vi "MoD Main-Optimize - HPLC RedAm_72117.vi"() -> ()   [LabVIEW 2015]
uses:
  <vilib>/silver_ctls/ArrayMatrixCluster/Real Matrix NI_Silver.ctl
  <vilib>/ni845x/ni845x.llb/ni845xControl.ctl
  <vilib>/MakerHub/LINX/Public/Peripherals/Analog/Analog Read 1 Chan.vi
  <vilib>/MakerHub/LINX/Public/Peripherals/Analog/Analog Read N Chans.vi
  <vilib>/MakerHub/LINX/Public/Peripherals/Digital/Digital Write 1 Chan.vi
  <vilib>/MakerHub/LINX/Private/Local IO/LinxAnalogRead.vi
  <vilib>/MakerHub/LINX/Public/Utilities/Check Channel.vi
  <vilib>/MakerHub/LINX/Public/Peripherals/Digital/Digital Write N Chans.vi
  <vilib>/MakerHub/LINX/Private/Local IO/LinxDigitalWrite.vi
  <vilib>/addons/control/pid/pid.llb/PID Control Input Filter (DBL).vi
  <vilib>/MakerHub/LINX/Private/Utilties/Generate Error.vi
  <vilib>/addons/control/pid/autopid.llb/PID Online Autotuning (Relay Feedback).vi
  <vilib>/Analysis/Matrix/Numeric/Conversions/Array To Matrix - RA2.vi
  <vilib>/ni845x/ni845x.llb/NI-845x Close Device Reference.vi
  <vilib>/addons/control/pid/NI_PID_autopid.lvlib
  <vilib>/addons/control/pid/NI_PID_pid.lvlib
  <vilib>/Analysis/Matrix/NI_Matrix.lvlib
  <vilib>/MakerHub/LINX/LMH-LINX.lvlib
  <instrlib>/Harvard Apparatus PHD Ultra Series/Harvard Apparatus PHD Ultra Series.lvlib
panel:
  out "running?":bool=TRUE
  out "new_reactor_volume":bool[](array[boolean])
  out "new_reactor_length":bool[](array[boolean])
  out "Phase_Sensor_voltage":dbl
  out "P_tot":dbl
  out "pause for ms":bool=TRUE
  out "stop_xl_write":bool=TRUE
  out "Num_exp_till_pause":i32
  out "Syringe_pump?":bool=TRUE
  out "System Error":bool=TRUE
  out "error out":errorcluster
  out "Pump setpoint(ul/min) 6":dbl format="%#_13g"
  out "Pump setpoint(ul/min) 5":dbl format="%#_13g"
  out "Pump setpoint(ul/min) 4":dbl format="%#_13g"
  out "Pump setpoint(ul/min) 3":dbl format="%#_13g"
  out "Pump setpoint(ul/min) 2":dbl format="%#_13g"
  out "Pump setpoint(ul/min) 1":dbl format="%#_13g"
  out "Volume (ul) 5":dbl format="%#_13g"
  out "Volume (ul) 4":dbl format="%#_13g"
  out "Volume (ul) 3":dbl format="%#_13g"
  out "Volume (ul) 2":dbl format="%#_13g"
  out "Volume (ul) 1":dbl format="%#_13g"
  in  "tau 5":dbl format="%#_13g"
  out "tau 4":dbl format="%#_13g"
  out "tau 3":dbl format="%#_13g"
  out "tau 2":dbl format="%#_13g"
  out "tau 1":dbl format="%#_13g"
  out "Reactor Length":dbl format="%#_13g"
  out "Flowrate Sensor 2":dbl format="%#_13g"
  out "Flowrate Sensor 1":dbl format="%#_13g"
  out "Pressure 2":dbl format="%#_13g"
  out "Pressure 1":dbl format="%#_13g"
  out "Temperature Control 5":bool=TRUE
  out "Temperature Control 4":bool=TRUE
  out "Temperature Control 3":bool=TRUE
  out "Temperature Control 2":bool=TRUE
  out "Temperature Control 1":bool=TRUE
  out "Temperature SP 5":dbl format="%#_g'C"
  out "Temperature SP 4":dbl format="%#_g'C"
  out "Temperature SP 3":dbl format="%#_g'C"
  out "Temperature SP 2":dbl format="%#_g'C"
  out "Temperature SP 1":dbl format="%#_g'C"
  in  "Bay Temperature 5":dbl
  in  "SSR Duration 5":dbl
  in  "SSR Duration 4":dbl
  in  "SSR Duration 3":dbl
  in  "SSR Duration 2":dbl
  in  "SSR Duration 1":dbl
  in  "Total Product Amount":dbl=1.0 format="%#_gml"
  out "Setup Error":bool=TRUE
  out "Error Message":string
  out "ID CTR":i32
  in  "Tab Control":T1(tab)
  out "Reagent pic 5":picture
  in  "reagent name 5":string
  out "Reagent Pic 4":picture
  in  "reagent name 4":string="Acetic Acid"
  out "Reagent Pic 3":picture
  in  "reagent  name 3":string="NaBH3CN"
  in  "Product name":string
  in  "reagent name 1":string="cyclohexylamine"
  out "Reagent Pic 1":picture
  in  "Vr5":dbl=45.6036 format="%#_guL"
  in  "Vr4":dbl format="%#_guL"
  in  "Vr3":dbl=45.6036 format="%#_guL"
  in  "Vr2":dbl format="%#_guL"
  in  "Vr1":dbl format="%#_guL"
  in  "System decide help Button":bool
  in  "Reaction Scheme Confirm":bool
  in  "Synthesis Route Array":string[][](array[string])=[["cyclohexylamine", ".1", "PhB(OH)2", "", "", ""], ["aldehyde + STD", ".1", "-", "-", "-", "-"], ["NaBH3CN", ".4", "-", "-", "-", "-"], ["Acetic Acid", "1", "-", "-", "-", "-"], ["", "", "-", "-", "-", "-"], ["", "", "-", "-", "-", "-"]]
  in  "System decide help Button 2":bool
  out "Setup Confirm":bool=TRUE
  in  "BAY 1":u16(ring)=1 items=["               Bypass", "         Heated Reactor", "    Small Heated Reator", "         Cooled Reactor", "      Packed Bed Reactor", "          Photo Reactor", "             Separator"]
  in  "BAY 5":u16(ring) items=["               Bypass", "         Heated Reactor", "    Small Heated Reactor", "         Cooled Reactor", "     Packed Bed Reactor", "         Photo Reactor", "             Separator"]
  in  "BAY 4":u16(ring) items=["                Bypass", "         Heated Reactor", "    Small Heated Reactor", "         Cooled Reactor", "     Packed Bed Reactor", "         Photo Reactor", "             Separator"]
  in  "BAY 3":u16(ring)=1 items=["               Bypass", "         Heated Reactor", "    Small Heated Reactor", "         Cooled Reactor", "     Packed Bed Reactor", "          Photo Reactor", "             Separator"]
  in  "BAY 2":u16(ring) items=["               Bypass", "         Heated Reactor", "    Small Heated Reactor", "         Cooled Reactor", "      Packed Bed Reactor", "          Photo Reactor", "             Separator"]
  out "Reagent Pic 2":picture
  out "Product Pic":picture
  in  "reagent name 2":string="benzylaldehyde"
  in  "reagent name 6":string
  out "Reagent Pic 6":picture
  in  "System Parameters Help Button":bool
  out "Setup Confirm 2":bool
  in  "System Parameters Confirm Button":bool
  in  "Bay Parameters":T2={"Bay 1 "={"Pump 1 Flowrate"=0.0, "optimize_temp"=TRUE, "optimize_tau"=TRUE, "Run at set flowrate"=FALSE, "Pump 2 Flowrate"=0.0, "Temperature Params"=[40.0, 100.0, 100.0], "pump params 1"=[43.0, 429.0, 325.0], "pump params 2"=[43.0, 429.0, 325.0], "Temperature"=0.0, "Run at set temperature"=FALSE}, "Bay 2 "={"Pump 3 Flowrate"=0.0, "optimize_temp"=FALSE, "optimize_tau"=TRUE, "Run at set flowrate"=FALSE, "Temperature Params"=[40.0, 100.0, 100.0], "Resisdence time params"=[38.03, 347.0, 650.0], "pump_at_ratio"=TRUE, "pump_num_ratio"=0.475, "Temperature"=0.0, "Run at set temperature"=FALSE}, "Bay 3 "={"Pump 4 Flowrate"=100.0, "optimize_temp"=FALSE, "optimize_tau"=FALSE, "Run at set flowrate"=FALSE, "Temperature Params"=[40.0, 100.0, 100.0], "Resisdence time params"=[3.8, 34.7, 0.0], "pump_at_ratio"=TRUE, "pump_num_ratio"=0.2, "Temperature "=100.0, "Run at set temperature"=TRUE}, "Bay 4 "={"Pump 5 Flowrate"=40.0, "Run at set flowrate"=FALSE, "optimize_temp"=FALSE, "optimize_tau"=FALSE, "Resisdence time params"=[10.0, 50.0, 225.0], "Temperature Params"=[40.0, 100.0, 80.0], "pump_at_ratio"=FALSE, "pump_num_ratio"=1.0, "Temperature"=0.0, "Run at set temperature"=FALSE}, "Bay 5 "={"Pump 6 Flowrate"=0.0, "Run at set flowrate"=FALSE, "optimize_temp"=FALSE, "optimize_tau"=FALSE, "Resisdence time params"=[1.0, 5.0, 0.0], "Temperature Params"=[0.0, 0.0, 0.0], "pump_at_ratio"=FALSE, "pump_num_ratio"=0.5, "Temperature"=0.0, "Run at set temperature"=FALSE}, "Excel File Name"="C:\\Users\\HPLC\\Dropbox (MIT)\\MoD Files\\Data\\RedAmin072117", "hplc File Name"="C:\\Chem32\\1\\Data\\MOD", "Matlab File"="C:\\Users\\HPLC\\Dropbox (MIT)\\MoD Files\\Data\\RedAmin072117", "Syringe for Pump 2?"=FALSE, "Num_conditons_per_wait"=2.0, "Continue from previous optimization?"=FALSE, "Total Number of Experiments 2"=15.0, "Hplc Wait time(min)"=10.0, "increas_decrease_hplc_peak"=TRUE, "Internal Standard?"=TRUE, "ISTD start"=8.0, "ISTD end"=10.0, "hplc_start"=1.75, "hplc_end"=3.0, "throughput_yield"=TRUE} {"Hplc Wait time(min)" format="%#_13g"; "Bay 5"."Temperature Params" format="%#_g'C"; "Bay 4"."Temperature Params" format="%#_g'C"; "Bay 3"."Temperature Params" format="%#_g'C"; "Bay 2"."Temperature Params" format="%#_g'C"; "Bay 1"."Temperature Params" format="%#_g'C"}
  out "System Confirm Not Clicked":string
  out "best_exp_num":dbl=1.0
  out "temperature_best":dbl[](array[numeric])
  out "Flowrates(ul/min)_best":dbl[](array[numeric])
  out "System Status":u16(ring)=2 caption="Sy" items=["System  Error", "System Running", "System Standby"]
  out "Current Experiment":dbl=1.0
  out "Total Number of Experiments":dbl=33.0
  out "Phase Sensor Chart":T3(graph)
  out "HPLC Analysis":bool
  out "Equlibrating Temperature":bool
  out "Flushing System":bool
  out "Calculate condition":bool
  out "Temperature 5":dbl format="%#_g'C"
  out "Temperature 4":dbl format="%#_g'C"
  out "Temperature 3":dbl format="%#_g'C"
  out "Temperature 2":dbl format="%#_g'C"
  out "Temperature 1":dbl format="%#_g'C"
  out "Flowrate Chart":T4(graph)
  out "Teperature Chart":T3(graph)
  out "Pump Setpoints Chart":T3(graph)
  out "Pressure Chart":T3(graph)
  out "Optimization_loop_index":i32
  out "curr_wait_time":dbl
  out "total_flush_time":dbl
  out "Temp SS? 5":bool=TRUE
  out "Temp SS? 4":bool=TRUE
  out "Temp SS? 3":bool=TRUE
  out "Temp SS? 2":bool=TRUE
  out "Temp SS? 1":bool=TRUE
  out "System Flushed?":bool
  out "stop_button clicked":bool
  out "experiment history":T5
  in  "Number of System Flushes per condtion":dbl=2.5
  in  "calculate volume 3":bool
  in  "calculate volume 2":bool=TRUE
  in  "calculate volume 1":bool=TRUE
  in  "calculate volume 4":bool=TRUE
  in  "calculate volume 5":bool
  in  "Extra system dead volume":dbl format="%#_gul"
  in  "new reactor length? 1":bool
  in  "tube_length(in)":dbl[](array[numeric])=[188.0, 188.0, 10.0, 10.0, 10.0]
  out "Pause Before Analysis":bool
  out "Chiller COMM Port":bool
  out "Arduino COMM Port 2":bool
  out "Temperature Sensor COMM Port":bool
  out "Flow Rate":bool
  out "Pressure":bool
  out "Pump COMM Port":bool
  in  "COMM Port :: Milligat Pumps":refnum<visa-resource-name>="COM10"
  in  "Arduino COMM Port":refnum<visa-resource-name>="COM3"
  in  "Sample Valve COMM::Port":refnum<visa-resource-name>="COM6"
  in  "COMM Port:: Harvard Syringe Pump":refnum<visa-resource-name>="COM5"
  in  "tube_id(in)":enum16{".01", ".02", ".03", ".04"}[](array[ring])=[enum.".03", enum.".03", enum.".03", enum.".03", enum.".03"]
  out "Total System Resisdence Time(min)":dbl
  in  "Debug_run_button":bool
  in  "new reactor length? 2":bool=TRUE
  in  "new reactor length? 3":bool
  in  "new reactor length? 4":bool
  in  "new reactor length? 5":bool
  in  "IR Sensor Device":T6="USB0::0x3923::0x7514::01B3FF21::RAW"
  out "Stop":bool=TRUE
  in  "Run_Stop_cluster":T7
  # "Molecules on Demand"
  # "Synthetic Route"
  # "5"
  # "6"
  # "4"
  # "Product"
  # "1"
  # "2"
  # "3"
  # "Reagent List"
  # "Concentration(M)"
  # "Molecule"
  # "1"
  # "1"
  # "2"
  # "2"
  # "3"
  # "3"
  # "4"
  # "4"
  # "5"
  # "6"
  # "5"
  # "6"
  # "Product"
  # "Reactor Volume:"
  # "Optimization Parameters"
  # "Pause after"
  # "Experiments"
  # "Optimize for"
  # "to"
  # "of HPLC Peak from"
  # "from"
  # "to"
  # "min"
  # "min"
  # "HPLC runtime"
  # "# Iterations"
  # "Reporting"
  # "Excel Output File Name"
  # "HPLC File Path"
  # "MATLAB File Path"
  # "Temperature"
  # "Flowrate(ul/min)"
  # "Lower Bound"
  # "Upper Bound"
  # "Optimize?"
  # "-or-"
  # "Run at"
  # "times incoming flow"
  # "Setpoint"
  # "Temperature"
  # "Flowrate(ul/min)"
  # "Lower Bound"
  # "Upper Bound"
  # "Optimize?"
  # "-or-"
  # "Run at"
  # "times incoming flow"
  # "Setpoint"
  # "Temperature"
  # "Flowrate(ul/min)"
  # "Lower Bound"
  # "Upper Bound"
  # "Optimize?"
  # "-or-"
  # "Run at"
  # "times incoming flow"
  # "Setpoint"
  # "Temperature"
  # "Flowrate 3 (ul/min)"
  # "Lower Bound"
  # "Upper Bound"
  # "Optimize?"
  # "-or-"
  # "Run at"
  # "times incoming flow"
  # "Setpoint"
  # "Temperature"
  # "Flowrate 1(ul/min)"
  # "Flowrate 2(ul/min)"
  # "Lower Bound"
  # "Upper Bound"
  # "Optimize?"
  # "Setpoint"
  # "Pressure (psi)"
  # "System Status"
  # "Temperature('C)"
  # "BAY"
  # "1"
  # "2"
  # "3"
  # "4"
  # "5"
  # "Pump Flowrate Setpoint(ul/min)"
  # "Flowrate (ul/min)"
  # "Phase Sensor"
  # "Current Experiment"
  # "Temperature('C)"
  # "Flowrate(ul/min)"
  # "Exp"
  # "Current Best Condition"
  # "Time to reach steady state:"
  # "Current Wait Time:"
  # "Experimental Steps"
  # "Calculated New Conditions"
  # "Steady State"
  # "Analyzed HPLC"
  # "Equilibrated Temperature"
  # "Tube Length (cm)"
  # "Bay"
  # "Tube ID (in)"
  # "Calculate Volume"
  # "Use new tube length"
  # "1."
  # "2."
  # "3."
  # "4."
  # "5."
  # "Reactor Lengths\n*Heated Reactor - 188cm * Small Reactor - 99cm * Bypass - 10cm * Separator - *"
  # "All Experimental Data"
  # "P1"
  # "P2"
  # "P3"
  # "P4"
  # "P5"
  # "P6"
  # "T1"
  # "T2"
  # "T3"
  # "T4"
  # "T5"
  # "Obj_fun"
  # "HPLC_Data"
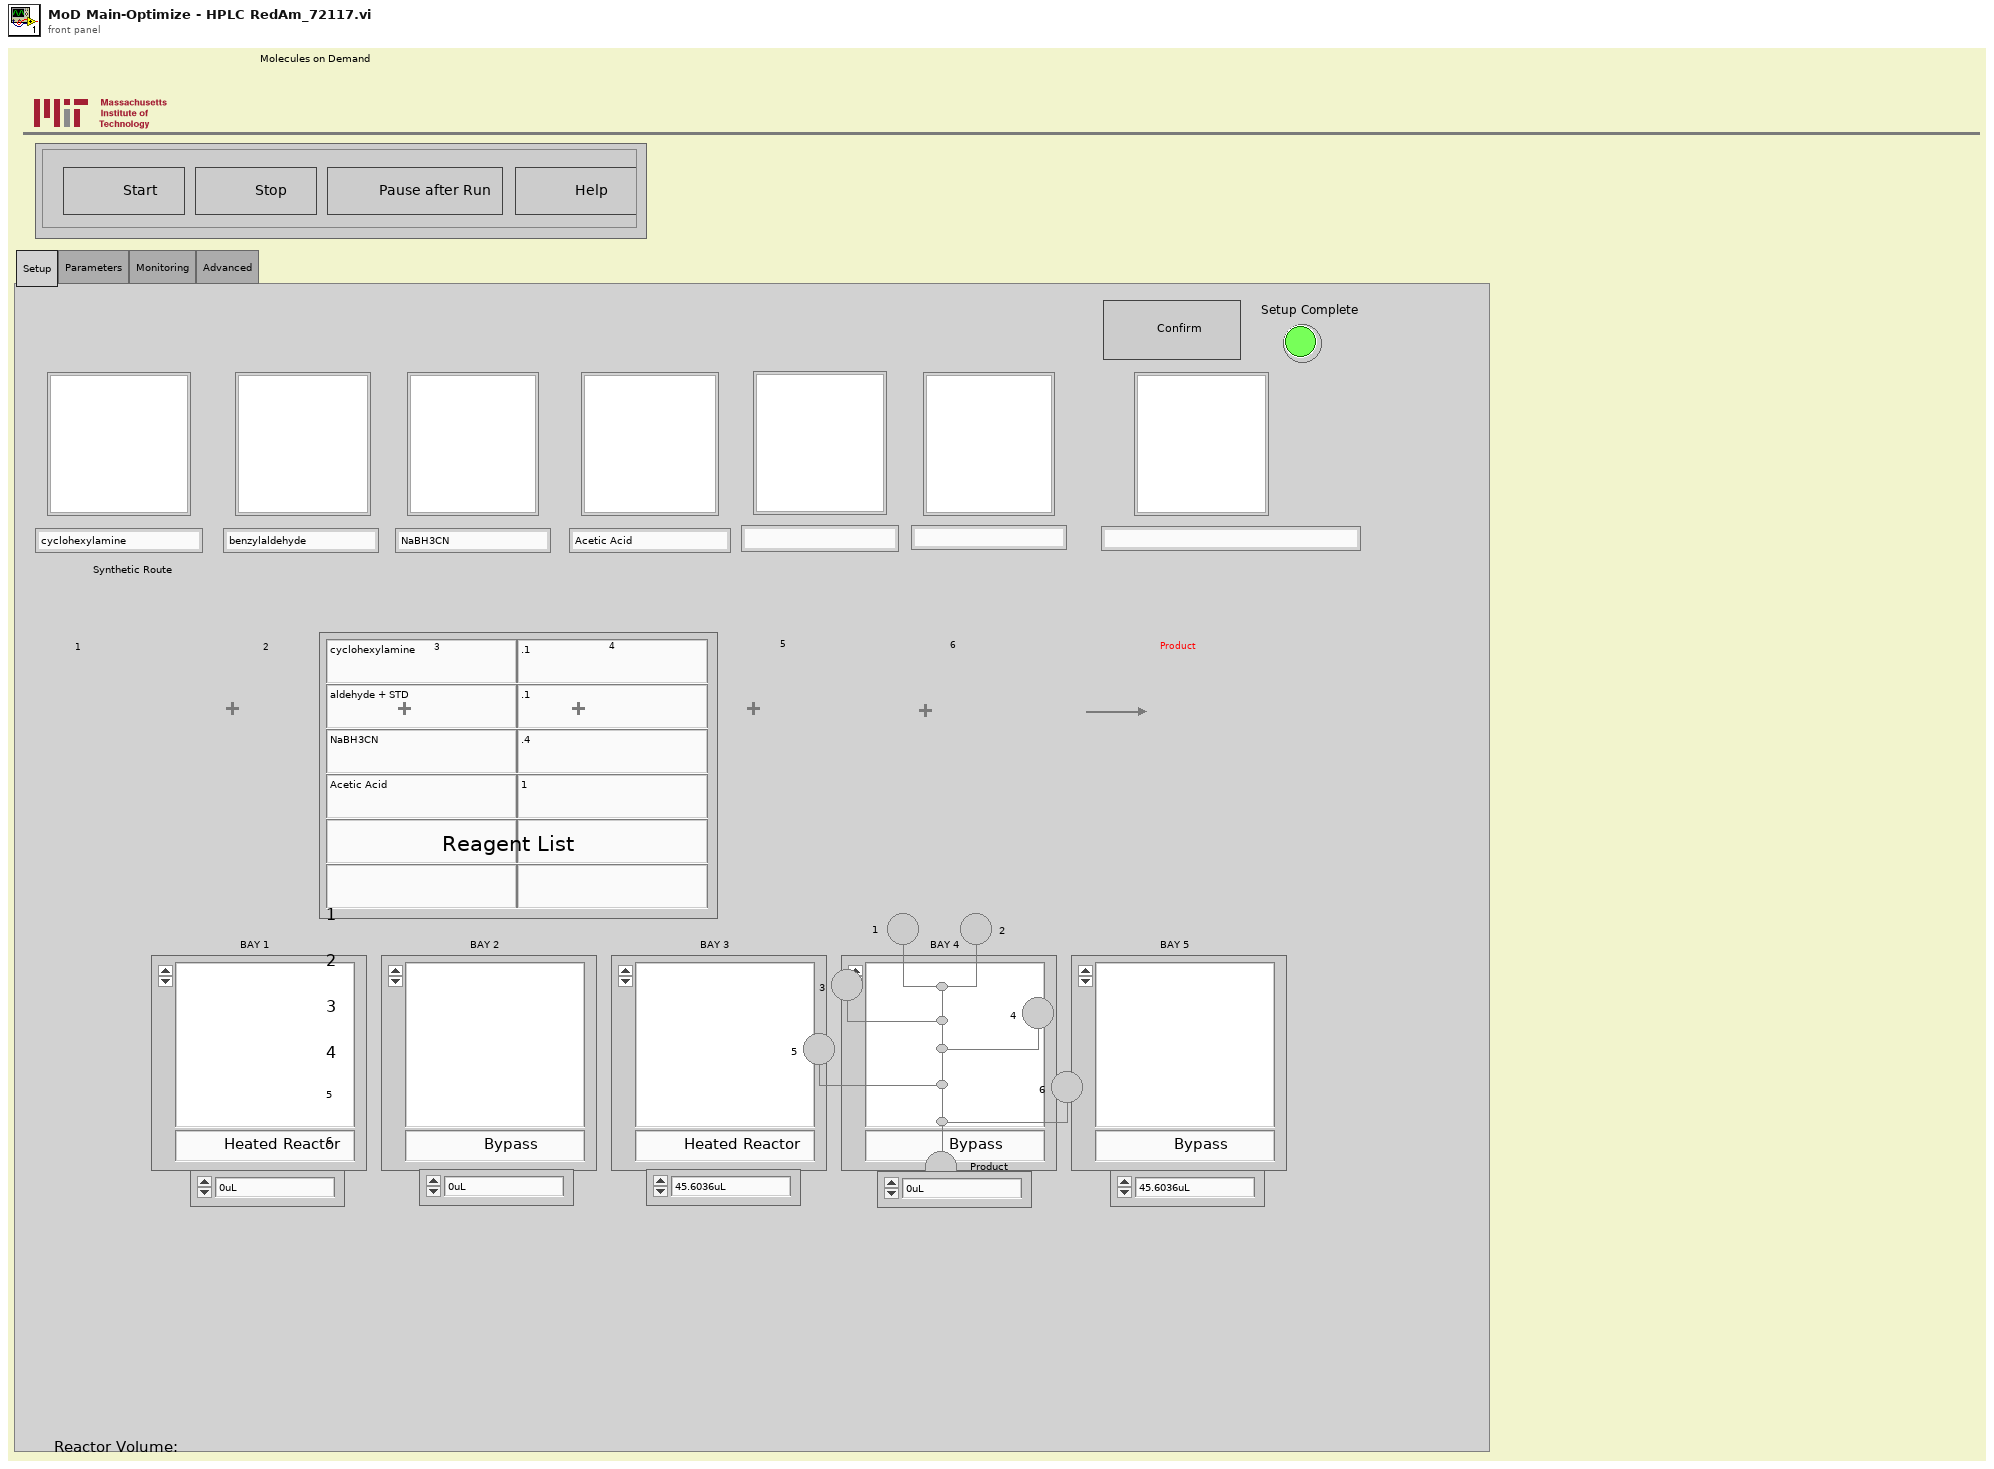
[diagram p1: front panel]
types:
  T1 = enum32{"Setup", "Parameters", "Monitoring", "Advanced"}
  T2 = cluster{"Bay 1 ":cluster{"Pump 1 Flowrate":dbl, "optimize_temp":bool, "optimize_tau":bool, "Run at set flowrate":bool, "Pump 2 Flowrate":dbl, "Temperature Params":dbl[], "pump params 1":dbl[], "pump params 2":dbl[], "Temperature":dbl, "Run at set temperature":bool}, "Bay 2 ":cluster{"Pump 3 Flowrate":dbl, "optimize_temp":bool, "optimize_tau":bool, "Run at set flowrate":bool, "Temperature Params":dbl[], "Resisdence time params":dbl[], "pump_at_ratio":bool, "pump_num_ratio":dbl, "Temperature":dbl, "Run at set temperature":bool}, "Bay 3 ":cluster{"Pump 4 Flowrate":dbl, "optimize_temp":bool, "optimize_tau":bool, "Run at set flowrate":bool, "Temperature Params":dbl[], "Resisdence time params":dbl[], "pump_at_ratio":bool, "pump_num_ratio":dbl, "Temperature ":dbl, "Run at set temperature":bool}, "Bay 4 ":cluster{"Pump 5 Flowrate":dbl, "Run at set flowrate":bool, "optimize_temp":bool, "optimize_tau":bool, "Resisdence time params":dbl[], "Temperature Params":dbl[], "pump_at_ratio":bool, "pump_num_ratio":dbl, "Temperature":dbl, "Run at set temperature":bool}, "Bay 5 ":cluster{"Pump 6 Flowrate":dbl, "Run at set flowrate":bool, "optimize_temp":bool, "optimize_tau":bool, "Resisdence time params":dbl[], "Temperature Params":dbl[], "pump_at_ratio":bool, "pump_num_ratio":dbl, "Temperature":dbl, "Run at set temperature":bool}, "Excel File Name":string, "hplc File Name":string, "Matlab File":string, "Syringe for Pump 2?":bool, "Num_conditons_per_wait":dbl, "Continue from previous optimization?":bool, "Total Number of Experiments 2":dbl, "Hplc Wait time(min)":dbl, "increas_decrease_hplc_peak":bool, "Internal Standard?":bool, "ISTD start":dbl, "ISTD end":dbl, "hplc_start":dbl, "hplc_end":dbl, "throughput_yield":bool}
  T3 = cluster{"[0]":dbl, "[1]":dbl, "[2]":dbl, "[3]":dbl, "[4]":dbl, "[5]":dbl, "[6]":dbl, "[7]":dbl, "[8]":dbl}
  T4 = cluster{"[0]":i32, "[1]":i32, "[2]":i32, "[3]":i32, "[4]":i32, "[5]":i32, "[6]":i32, "[7]":i32, "[8]":i32}
  T5 = typedef "Real Matrix NI_Silver.ctl" = dbl[][]
  T6 = typedef "ni845xControl.ctl" = refnum<k21>
  T7 = cluster{"Stop":bool, "Run":bool, "Stop Run Button":bool, "Help Button":bool}
  T8 = cluster{"Proportional gain Kc":dbl, "Integral time Ti (sec)":dbl, "Derivative time Ti (sec)":dbl}
  T9 = cluster{"type of controller":enum16{"P", "PI", "PID"}, "relay cycles":i32, "relay amplitude":dbl, "control specifications":enum16{"Fast", "Normal", "Slow"}, "PV noise level":dbl}
  T10 = typedef "LMH-LINX.lvlib/LINX Ref.ctl" = cluster{"IO":T11, "Interface":T12, "LINX Device Config":T13}
  T11 = typedef "LMH-LINX.lvlib/Platform.ctl" = enum16{"Remote", "Local"}
  T12 = typedef "LMH-LINX.lvlib/Interface.ctl" = enum16{"Serial", "TCP"}
  T13 = typedef "LMH-LINX.lvlib/Device.lvlib/LINX Device Config.ctl" = cluster{"Interface":T12, "COM Port":refnum<visa-resource-name>, "TCP Configuration":T14, "Device Family":u8, "Device ID":u8, "Device Name":string, "TCP Ref":refnum<k5>, "Channels":T15}
  T14 = typedef "LMH-LINX.lvlib/Device.lvlib/TCP Config.ctl" = cluster{"IP Address":string, "Port":u16}
  T15 = typedef "LMH-LINX.lvlib/Channels.ctl" = cluster{"DI":u8[], "DO":u8[], "AI":u8[], "AO":u8[], "PWM":u8[], "QE":u8[], "UART":u8[], "I2C 2":u8[], "SPI":u8[], "CAN":u8[], "Servo":u8[], "AI Ref (V)":dbl, "AI Resolution (Bits)":u8, "AO Ref (V)":dbl, "AO Resolution (Bits)":u8}
  T16 = typedef "imagedata.ctl" = cluster{"image type":i32, "image depth":i32, "image":u8[], "mask":u8[], "colors":u32[], "Rectangle":cluster{"left":i16, "top":i16, "right":i16, "bottom":i16}}
  T17 = cluster{"proportional gain (Kc)":dbl, "integral time (Ti, min)":dbl, "derivative time (Td, min)":dbl}
  T18 = typedef "NI_Matrix.lvlib/RealMatrix.ctl" = dbl[][]
  T19 = enum16{"Left Button", "Center Button", "Right Button", "Window Close"}
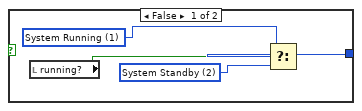
[diagram p3: hidden frame]
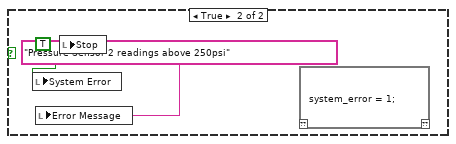
[diagram p4: hidden frame]
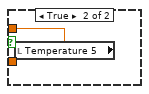
[diagram p6: hidden frame]
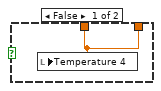
[diagram p7: hidden frame]
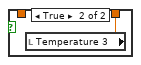
[diagram p8: hidden frame]
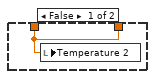
[diagram p9: hidden frame]
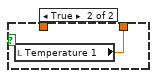
[diagram p10: hidden frame]
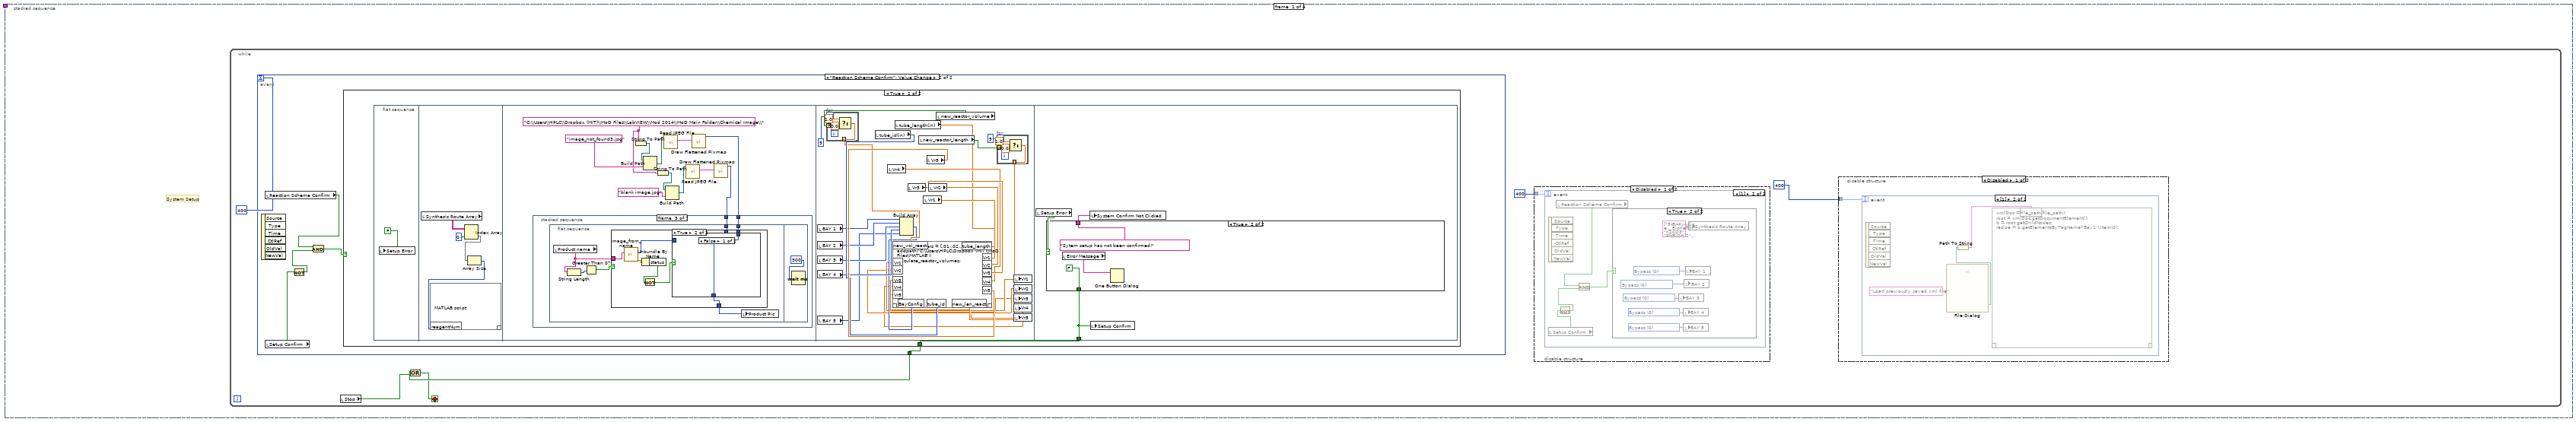
[diagram p11: hidden frame]
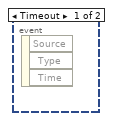
[diagram p12: hidden frame]
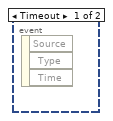
[diagram p14: hidden frame]
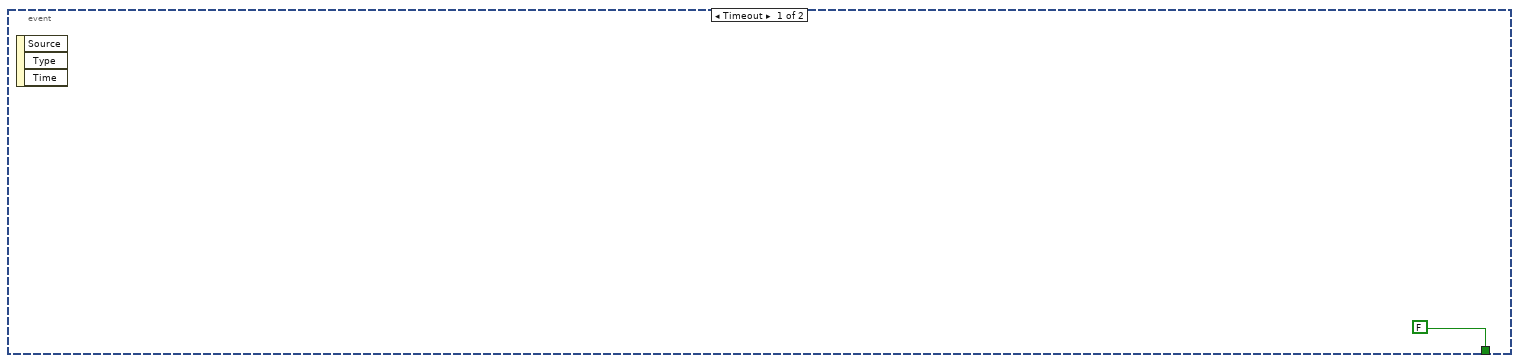
[diagram p17: hidden frame]
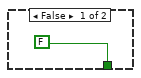
[diagram p18: hidden frame]
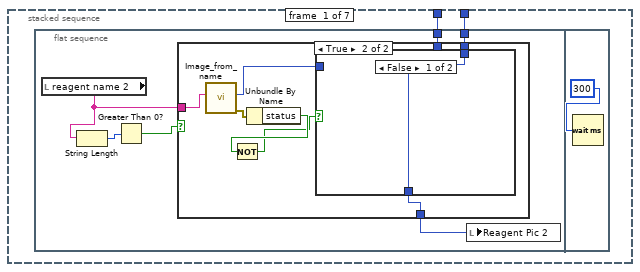
[diagram p19: hidden frame]
diagram:
  # "Assume User always uses the first bay first"
  n1 = flat-sequence {
    tunnel: ["COMM Port :: Milligat Pumps"] -> w9
    tunnel: ["Arduino COMM Port"] -> w8
    tunnel: [w11] -> w5
    tunnel: ["Bay Parameters"] -> w4
    tunnel: [w60] -> w10
    tunnel: w9 -> [w60]
    tunnel: w8 -> [w48]
    tunnel: [w54] -> w7
    tunnel: [w52] -> w6
    tunnel: w5 -> [w52]
    tunnel: w4 -> [w50]
    tunnel: [w47] -> w3
    tunnel: w10 -> [w66]
    tunnel: w7 -> [w65]
    tunnel: w6 -> [w63]
    tunnel: w3 -> [w61]
    tunnel: [w61] -> w1
    tunnel: [w1375] -> w2
    tunnel: w1 -> [w1375]
    tunnel: w2 -> [w1376]
    frame #0 {
      w36 = FALSE ("Equlibrating Temperature")
      n2 = script code="TempArr1=[23 23 23 23 23 23 23 23 23 23]';\nTempArr2=[23 23 23 23 23 23 23 23 23 23]';\nTempArr3=[23 23 23 23 23 23 23 23 23 23]';\nTempArr4=[23 23 23 23 23 23 23 23 23 23]';\nTempArr5=[23 23 23 23 23 23 23 23 23 23]';\ntemp_error1 =0;\ntemp_error2 =0;\ntemp_error3 =0;\ntemp_error4 =0;\ntemp_error5 =0;\ntemp_check1 = 0;\ntemp_check2 = 0;\ntemp_check3 = 0;\ntemp_check4 = 0;\ntemp_check5 = 0;\nT1=23;\nT2=23;\nT3=23;\nT4=23;\nT5=23;"() -> ()  [unwired: 1 in, 1 out]
      n3 = Build Array("calculate volume 1", "calculate volume 2", "calculate volume 3", "calculate volume 4", "calculate volume 5") -> (→"new_reactor_volume":bool[])
      n4 = Build Array("new reactor length? 1", "new reactor length? 2", "new reactor length? 3", "new reactor length? 4", "new reactor length? 5") -> (→"new_reactor_length":bool[])
      n5 = call <vilib>:"Initialize.vi"("VISA resource name"="COMM Port:: Harvard Syringe Pump") -> ("VISA resource name out"=w11:refnum<visa-resource-name>)  [unwired: 9 in, 1 out]
      "Stop" <- FALSE ("Stop")
      "ID CTR" <- 0
      "Setup Confirm" <- FALSE ("Setup Confirm")
      "Error Message" <- "System shutdown sucessfully. No errors to report." ("Error Message")
      "Setup Error" <- FALSE ("Setup Error")
      "Reactor Length" <- 10.5
      "System Error" <- FALSE ("System Error")
      "Num_exp_till_pause" <- 0 ("Num_exp_till_pause")
      "Equlibrating Temperature" <- w36
      "Calculate condition" <- w36
      "Flushing System" <- w36
      "HPLC Analysis" <- w36
      "stop_xl_write" <- FALSE ("stop_xl_write")
      "Pump setpoint(ul/min) 1" <- 0.0 ("Pump setpoint(ul/min) 1")
      "Pump setpoint(ul/min) 2" <- 0.0 ("Pump setpoint(ul/min) 2")
      "Pump setpoint(ul/min) 4" <- 0.0 ("Pump setpoint(ul/min) 4")
      "Pump setpoint(ul/min) 6" <- 0.0 ("Pump setpoint(ul/min) 6")
      "Pump setpoint(ul/min) 3" <- 0.0 ("Pump setpoint(ul/min) 3")
      "Pump setpoint(ul/min) 5" <- 0.0 ("Pump setpoint(ul/min) 5")
      "pause for ms" <- FALSE ("pause for ms")
      "Setup Confirm 2" <- FALSE ("Setup Confirm 2")
      "running?" <- FALSE ("running?")
    }
    frame #1 {
      w49 = FALSE
      w59 = 23
      (unwired) path "C:/Users/User1/Documents/Lab/MoD/Images"
      n6 = disable-structure shown="Disabled" {
        frame Disabled {
          n7 = local read "BAY 2"() -> ()  [unwired: 1 out]
          n8 = local read "BAY 3"() -> ()  [unwired: 1 out]
          n9 = local read "BAY 4"() -> ()  [unwired: 1 out]
          n10 = local read "BAY 5"() -> ()  [unwired: 1 out]
          n11 = local read "BAY 1"() -> ()  [unwired: 1 out]
        }
        frame Enabled {
        }
      }
      n12 = local write "Debug_run_button"(TRUE) -> ()
      n13 = call <vilib>:"Initialize.vi"("Serial Port"=w48) -> ("LINX Resource"=w47:T10)  [unwired: 8 in, 2 out]
      n14 = local write "System Parameters Confirm Button"(w49) -> ()
      n15 = local write "Setup Confirm 2"(w49) -> ()
      n16 = Unbundle By Name(w50) -> ("Syringe for Pump 2?"=→"Syringe_pump?":bool)
      n17 = local write "Temperature 1"(w59) -> ()
      n18 = local write "Temperature 2"(w59) -> ()
      n19 = local write "Temperature 3"(w59) -> ()
      n20 = local write "Temperature 4"(w59) -> ()
      n21 = local write "Temperature 5"(w59) -> ()
      n22 = local write "Temperature SP 1"(w59) -> ()
      n23 = local write "Temperature SP 2"(w59) -> ()
      n24 = local write "Temperature SP 3"(w59) -> ()
      n25 = local write "Temperature SP 4"(w59) -> ()
      n26 = local write "Temperature SP 5"(w59) -> ()
      n27 = Current VI's Path() -> (path=w58:path)
      n28 = Strip Path(path=w58) -> (stripped path=w56:path)  [unwired: 1 out]
      n29 = Strip Path(path=w56) -> (stripped path=w55:path)  [unwired: 1 out]
      n30 = Build Path(base path=w55, name or relative path="MATLAB") -> (appended path=w54:path)
    }
    frame #2 {
      # "Main Help Dialog Popup"
      n31 = while {
        stop <- w1369 stop-if-true
        n32 = event shown="[6] \"Run_Stop_cluster.Run\": Value Change" {
          selector: _ -> [_ _ _ _ _ _ _]
          dyn-events: _ -> [_ _ _ _ _ _ _]
          timeout: 100 -> [_ _ _ _ _ _ _]
          event Timeout {
            n33 = event-data() -> ()  [unwired: 1 in, 3 out]
          }
          event "Run_Stop_cluster.Help Button": Value Change {
            n34 = local read "Run_Stop_cluster"() -> (w1372:T7)
            n35 = event-data() -> ()  [unwired: 1 in, 4 out]
            n36 = Unbundle By Name(w1372) -> ("Help Button"=w1371:bool)
            n37 = case shown="True" w1371 {
              frame False {
              }
              frame True {
                n38 = call "help.vi"() -> ()  [unwired: 11 in]
              }
            }
          }
          event "System decide help Button": Value Change {
            n39 = event-data() -> ()  [unwired: 1 in, 5 out]
            n40 = call "help_synthesis_man-auto_instructions.vi"() -> ()  [unwired: 12 in]
          }
          event "System Parameters Help Button": Value Change {
            n41 = event-data() -> ()  [unwired: 1 in, 5 out]
            n42 = call "help_parameters_setup.vi"() -> ()  [unwired: 12 in]
          }
          event "System decide help Button 2": Value Change {
            n43 = event-data() -> ()  [unwired: 1 in, 5 out]
            n44 = call "help_synthesis_route_instructions.vi"() -> ()  [unwired: 12 in]
          }
          event "Run_Stop_cluster.Stop": Value Change {
            n45 = event-data() -> ()  [unwired: 1 in, 5 out]
            n46 = local write "Stop"(TRUE) -> ()
          }
          event "Run_Stop_cluster.Run": Value Change {
            n47 = event-data() -> ()  [unwired: 1 in, 5 out]
            n48 = local write "running?"(TRUE) -> ()
          }
        }
        n49 = local read "Stop"() -> (w1369:bool)
      }
      n50 = stacked-sequence {
        tunnel: w66 -> [_ _ _ _]
        tunnel: w65 -> [_ w425 _ _]
        tunnel: w63 -> [_ _ _ w592]
        tunnel: w61 -> [_ _ _ w590]
        frame #0 {
          # "System Setup"
          n51 = while {
            stop <- w200 stop-if-true
            n52 = event shown="[1] \"Reaction Scheme Confirm\": Value Change" {
              selector: _ -> [_ _]
              dyn-events: _ -> [_ _]
              timeout: 400 -> [_ _]
              tunnel: [FALSE w220] -> w202
              event Timeout {
                n53 = event-data() -> ()  [unwired: 1 in, 3 out]
              }
              event "Reaction Scheme Confirm": Value Change {
                n54 = event-data() -> ()  [unwired: 1 in, 6 out]
                n55 = local read "Reaction Scheme Confirm"() -> (w224:bool)
                n56 = local read "Setup Confirm"() -> (w222:bool)
                n57 = Not(x=w222) -> (.not. x?=w221:bool)
                n58 = And(x=w224, y=w221) -> (x .and. y?=w223:bool)
                n59 = case shown="True" w223 {
                  tunnel: [FALSE w226] -> w220
                  frame False {
                  }
                  frame True {
                    n60 = flat-sequence {
                      tunnel: [w415] -> w226
                      frame #0 {
                        n61 = local write "Setup Error"(FALSE) -> ()
                      }
                      frame #1 {
                        n62 = local read "Synthesis Route Array"() -> (w230:string[][])
                        n63 = Index Array(array=w230, index (col)=0 ("disabled index (col)")) -> (element=w228:string[])  [unwired: 1 in]
                        n64 = Array Size(array=w228) -> (size(s)=w231:i32)
                        n65 = script code="MATLAB script"("reagentNum"=w231) -> ()  [unwired: 1 in, 1 out]
                      }
                      frame #2 {
                        w234 = "C:\\Users\\HPLC\\Dropbox (MIT)\\MoD Files\\LabVIEW\\Mod 2014\\MoD Main Folder\\Chemical Image\\" ("string")
                        n66 = String To Path(string=w234) -> (path=w240:path)
                        n67 = Build Path(base path=w240, name or relative path="image_not_found3.jpg") -> (appended path=w239:path)
                        n68 = String To Path(string=w234) -> (path=w237:path)
                        n69 = call <vilib>:"Read JPEG File.vi"("path to JPEG file"=w239) -> ("image data"=w242:T16)  [unwired: 1 in, 9 out]
                        n70 = Build Path(base path=w237, name or relative path="blank image.jpg") -> (appended path=w235:path)
                        n71 = call <vilib>:"Read JPEG File.vi"("path to JPEG file"=w235) -> ("image data"=w238:T16)  [unwired: 1 in, 9 out]
                        n72 = call <vilib>:"Draw Flattened Pixmap.vi"("image data"=w242) -> ("new picture"=w233:picture)  [unwired: 3 in, 5 out]
                        n73 = call <vilib>:"Draw Flattened Pixmap.vi"("image data"=w238) -> ("new picture"=w232:picture)  [unwired: 3 in, 5 out]
                        n74 = stacked-sequence {
                          tunnel: w233 -> [w244 w264 w284 w304 w324 w343 w363]
                          tunnel: w232 -> [w243 w263 w283 w303 w323 w344 w364]
                          frame #0 {
                            n75 = flat-sequence {
                              tunnel: w244 -> [w250]
                              tunnel: w243 -> [w248]
                              frame #0 {
                                n76 = local read "reagent name 2"() -> (w246:string)
                                n77 = String Length(string=w246) -> (length=w249:i32)
                                n78 = Greater Than 0?(x=w249) -> (x > 0?=w247:bool)
                                n79 = case shown="True" w247 {
                                tunnel: w250 -> [_ w256]
                                tunnel: w248 -> [w251 _]
                                tunnel: [w251 w255] -> w245
                                tunnel: w246 -> [_ w254]
                                frame False {
                                }
                                frame True {
                                n80 = call "Image_from_name.vi"("Chemical Name"=w254) -> ("error out"=w257:errorcluster, "Downloaded Picture"=w258:picture)  [unwired: 8 in, 1 out]
                                n81 = Unbundle By Name(w257) -> ("status"=w253:bool)
                                n82 = Not(x=w253) -> (.not. x?=w252:bool)
                                n83 = case shown="False" w252 {
                                tunnel: w258 -> [_ w261]
                                tunnel: [w259 w260] -> w255
                                tunnel: w256 -> [w259 _]
                                frame False {
                                }
                                frame True {
                                n84 = call <vilib>:"Draw Flattened Pixmap.vi"("picture"=w261) -> ("new picture"=w260:picture)  [unwired: 8 in]
                                }
                                }
                                }
                                }
                                n85 = local write "Reagent Pic 2"(w245) -> ()
                              }
                              frame #1 {
                                n86 = Wait (ms)(milliseconds to wait=300) -> ()  [unwired: 1 out]
                              }
                            }
                          }
                          frame #1 {
                            n87 = flat-sequence {
                              tunnel: w264 -> [w270]
                              tunnel: w263 -> [w268]
                              frame #0 {
                                n88 = local read "reagent name 1"() -> (w265:string)
                                n89 = String Length(string=w265) -> (length=w269:i32)
                                n90 = Greater Than 0?(x=w269) -> (x > 0?=w267:bool)
                                n91 = case shown="True" w267 {
                                tunnel: w270 -> [_ w276]
                                tunnel: w268 -> [w271 _]
                                tunnel: [w271 w275] -> w266
                                tunnel: w265 -> [_ w274]
                                frame False {
                                }
                                frame True {
                                n92 = call "Image_from_name.vi"("Chemical Name"=w274) -> ("error out"=w277:errorcluster, "Downloaded Picture"=w278:picture)  [unwired: 8 in, 1 out]
                                n93 = Unbundle By Name(w277) -> ("status"=w273:bool)
                                n94 = Not(x=w273) -> (.not. x?=w272:bool)
                                n95 = case shown="True" w272 {
                                tunnel: w278 -> [_ w281]
                                tunnel: [w279 w280] -> w275
                                tunnel: w276 -> [w279 _]
                                frame False {
                                }
                                frame True {
                                n96 = call <vilib>:"Draw Flattened Pixmap.vi"("picture"=w281) -> ("new picture"=w280:picture)  [unwired: 8 in]
                                }
                                }
                                }
                                }
                                n97 = local write "Reagent Pic 1"(w266) -> ()
                              }
                              frame #1 {
                                n98 = Wait (ms)(milliseconds to wait=300) -> ()  [unwired: 1 out]
                              }
                            }
                          }
                          frame #2 {
                            n99 = flat-sequence {
                              tunnel: w284 -> [w290]
                              tunnel: w283 -> [w288]
                              frame #0 {
                                n100 = local read "Product name"() -> (w285:string)
                                n101 = String Length(string=w285) -> (length=w289:i32)
                                n102 = Greater Than 0?(x=w289) -> (x > 0?=w287:bool)
                                n103 = case shown="True" w287 {
                                tunnel: w290 -> [_ w296]
                                tunnel: w288 -> [w291 _]
                                tunnel: [w291 w295] -> w286
                                tunnel: w285 -> [_ w294]
                                frame False {
                                }
                                frame True {
                                n104 = call "Image_from_name.vi"("Chemical Name"=w294) -> ("error out"=w297:errorcluster, "Downloaded Picture"=w298:picture)  [unwired: 8 in, 1 out]
                                n105 = Unbundle By Name(w297) -> ("status"=w292:bool)
                                n106 = Not(x=w292) -> (.not. x?=w293:bool)
                                n107 = case shown="False" w293 {
                                tunnel: w298 -> [_ w301]
                                tunnel: [w299 w300] -> w295
                                tunnel: w296 -> [w299 _]
                                frame False {
                                }
                                frame True {
                                n108 = call <vilib>:"Draw Flattened Pixmap.vi"("picture"=w301) -> ("new picture"=w300:picture)  [unwired: 8 in]
                                }
                                }
                                }
                                }
                                n109 = local write "Product Pic"(w286) -> ()
                              }
                              frame #1 {
                                n110 = Wait (ms)(milliseconds to wait=300) -> ()  [unwired: 1 out]
                              }
                            }
                          }
                          frame #3 {
                            n111 = flat-sequence {
                              tunnel: w304 -> [w310]
                              tunnel: w303 -> [w308]
                              frame #0 {
                                n112 = local read "reagent name 6"() -> (w305:string)
                                n113 = String Length(string=w305) -> (length=w309:i32)
                                n114 = Greater Than 0?(x=w309) -> (x > 0?=w307:bool)
                                n115 = case shown="True" w307 {
                                tunnel: w310 -> [_ w316]
                                tunnel: w308 -> [w311 _]
                                tunnel: [w311 w315] -> w306
                                tunnel: w305 -> [_ w314]
                                frame False {
                                }
                                frame True {
                                n116 = call "Image_from_name.vi"("Chemical Name"=w314) -> ("error out"=w317:errorcluster, "Downloaded Picture"=w318:picture)  [unwired: 8 in, 1 out]
                                n117 = Unbundle By Name(w317) -> ("status"=w312:bool)
                                n118 = Not(x=w312) -> (.not. x?=w313:bool)
                                n119 = case shown="False" w313 {
                                tunnel: w318 -> [_ w321]
                                tunnel: [w319 w320] -> w315
                                tunnel: w316 -> [w319 _]
                                frame False {
                                }
                                frame True {
                                n120 = call <vilib>:"Draw Flattened Pixmap.vi"("picture"=w321) -> ("new picture"=w320:picture)  [unwired: 8 in]
                                }
                                }
                                }
                                }
                                n121 = local write "Reagent Pic 6"(w306) -> ()
                              }
                              frame #1 {
                                n122 = Wait (ms)(milliseconds to wait=300) -> ()  [unwired: 1 out]
                              }
                            }
                          }
                          frame #4 {
                            n123 = flat-sequence {
                              tunnel: w324 -> [w330]
                              tunnel: w323 -> [w328]
                              frame #0 {
                                n124 = local read "reagent name 5"() -> (w325:string)
                                n125 = String Length(string=w325) -> (length=w329:i32)
                                n126 = Greater Than 0?(x=w329) -> (x > 0?=w327:bool)
                                n127 = case shown="True" w327 {
                                tunnel: w330 -> [_ w336]
                                tunnel: w328 -> [w331 _]
                                tunnel: [w331 w335] -> w326
                                tunnel: w325 -> [_ w334]
                                frame False {
                                }
                                frame True {
                                n128 = call "Image_from_name.vi"("Chemical Name"=w334) -> ("error out"=w337:errorcluster, "Downloaded Picture"=w338:picture)  [unwired: 8 in, 1 out]
                                n129 = Unbundle By Name(w337) -> ("status"=w332:bool)
                                n130 = Not(x=w332) -> (.not. x?=w333:bool)
                                n131 = case shown="False" w333 {
                                tunnel: w338 -> [_ w341]
                                tunnel: [w339 w340] -> w335
                                tunnel: w336 -> [w339 _]
                                frame False {
                                }
                                frame True {
                                n132 = call <vilib>:"Draw Flattened Pixmap.vi"("picture"=w341) -> ("new picture"=w340:picture)  [unwired: 8 in]
                                }
                                }
                                }
                                }
                                n133 = local write "Reagent pic 5"(w326) -> ()
                              }
                              frame #1 {
                                n134 = Wait (ms)(milliseconds to wait=300) -> ()  [unwired: 1 out]
                              }
                            }
                          }
                          frame #5 {
                            n135 = flat-sequence {
                              tunnel: w344 -> [w348]
                              tunnel: w343 -> [w347]
                              frame #0 {
                                n136 = local read "reagent name 4"() -> (w345:string)
                                n137 = String Length(string=w345) -> (length=w350:i32)
                                n138 = Greater Than 0?(x=w350) -> (x > 0?=w349:bool)
                                n139 = case shown="True" w349 {
                                tunnel: w347 -> [_ w356]
                                tunnel: w348 -> [w351 _]
                                tunnel: [w351 w355] -> w346
                                tunnel: w345 -> [_ w354]
                                frame False {
                                }
                                frame True {
                                n140 = call "Image_from_name.vi"("Chemical Name"=w354) -> ("error out"=w357:errorcluster, "Downloaded Picture"=w358:picture)  [unwired: 8 in, 1 out]
                                n141 = Unbundle By Name(w357) -> ("status"=w352:bool)
                                n142 = Not(x=w352) -> (.not. x?=w353:bool)
                                n143 = case shown="False" w353 {
                                tunnel: w358 -> [_ w361]
                                tunnel: [w359 w360] -> w355
                                tunnel: w356 -> [w359 _]
                                frame False {
                                }
                                frame True {
                                n144 = call <vilib>:"Draw Flattened Pixmap.vi"("picture"=w361) -> ("new picture"=w360:picture)  [unwired: 8 in]
                                }
                                }
                                }
                                }
                                n145 = local write "Reagent Pic 4"(w346) -> ()
                              }
                              frame #1 {
                                n146 = Wait (ms)(milliseconds to wait=300) -> ()  [unwired: 1 out]
                              }
                            }
                          }
                          frame #6 {
                            n147 = flat-sequence {
                              tunnel: w364 -> [w368]
                              tunnel: w363 -> [w367]
                              frame #0 {
                                n148 = local read "reagent  name 3"() -> (w365:string)
                                n149 = String Length(string=w365) -> (length=w370:i32)
                                n150 = Greater Than 0?(x=w370) -> (x > 0?=w369:bool)
                                n151 = case shown="True" w369 {
                                tunnel: w367 -> [_ w376]
                                tunnel: w368 -> [w371 _]
                                tunnel: [w371 w375] -> w366
                                tunnel: w365 -> [_ w374]
                                frame False {
                                }
                                frame True {
                                n152 = call "Image_from_name.vi"("Chemical Name"=w374) -> ("error out"=w377:errorcluster, "Downloaded Picture"=w378:picture)  [unwired: 8 in, 1 out]
                                n153 = Unbundle By Name(w377) -> ("status"=w372:bool)
                                n154 = Not(x=w372) -> (.not. x?=w373:bool)
                                n155 = case shown="False" w373 {
                                tunnel: w378 -> [_ w381]
                                tunnel: [w379 w380] -> w375
                                tunnel: w376 -> [w379 _]
                                frame False {
                                }
                                frame True {
                                n156 = call <vilib>:"Draw Flattened Pixmap.vi"("picture"=w381) -> ("new picture"=w380:picture)  [unwired: 8 in]
                                }
                                }
                                }
                                }
                                n157 = local write "Reagent Pic 3"(w366) -> ()
                              }
                              frame #1 {
                                n158 = Wait (ms)(milliseconds to wait=300) -> ()  [unwired: 1 out]
                              }
                            }
                          }
                        }
                      }
                      frame #3 {
                        n159 = local read "BAY 1"() -> (w393:u16)
                        n160 = local read "BAY 2"() -> (w392:u16)
                        n161 = local read "BAY 3"() -> (w391:u16)
                        n162 = local read "BAY 4"() -> (w390:u16)
                        n163 = local read "BAY 5"() -> (w389:u16)
                        n164 = local read "tube_id(in)"() -> (w400:enum16{".01", ".02", ".03", ".04"}[])
                        n165 = local read "Vr4"() -> (w403:dbl)
                        n166 = local read "tube_length(in)"() -> (w401:dbl[])
                        n167 = Build Array(w393, w392, w391, w390, w389) -> (w388:u16[])
                        n168 = local read "Vr3"() -> (w404:dbl)
                        n169 = local read "new_reactor_length"() -> (w398:bool[])
                        n170 = local read "Vr1"() -> (w406:dbl)
                        n171 = local read "Vr5"() -> (w402:dbl)
                        n172 = local read "Vr2"() -> (w405:dbl)
                        n173 = local read "new_reactor_volume"() -> (w396:bool[])
                        n174 = for {
                          N: 5 -> [_]
                          tunnel: w396 -> [w410] mode=indexing
                          tunnel: [w407] -> w394 mode=indexing
                          n175 = Select(t=1.0, s=w410, f=0.0) -> (s? t:f=w407:dbl)
                        }
                        n176 = for {
                          N: 5 -> [_]
                          tunnel: w398 -> [w414] mode=indexing
                          tunnel: [w411] -> w397 mode=indexing
                          n177 = Select(t=1.0, s=w414, f=0.0) -> (s? t:f=w411:dbl)
                        }
                        n178 = script code="tube_diameters = [.01,.02,.03,.04];\naddpath('C:\\Users\\HPLC\\Dropbox (MIT)\\MoD Files\\MATLAB');\ncalculate_reactor_volumes;"("BayConfig"=w388, "Vr1"=w406, "Vr2"=w405, "Vr3"=w404, "Vr4"=w403, "Vr5"=w402, "tube_length"=w401, "tube_id"=w400, "new_len_react"=w397, "new_vol_react"=w394) -> ("Vr1"=w387:dbl, "Vr2"=w386:dbl, "Vr3"=w385:dbl, "Vr4"=w384:dbl, "Vr5"=w383:dbl)  [unwired: 1 in, 1 out]
                        n179 = local write "Vr1"(w387) -> ()
                        n180 = local write "Vr2"(w386) -> ()
                        n181 = local write "Vr3"(w385) -> ()
                        n182 = local write "Vr4"(w384) -> ()
                        n183 = local write "Vr5"(w383) -> ()
                      }
                      frame #4 {
                        n184 = local read "Setup Error"() -> (w417:bool)
                        n185 = case shown="True" w417 {
                          tunnel: [TRUE FALSE] -> w415
                          tunnel: ["" "Sytem setup has not been confirmed!"] -> w416
                          frame False {
                          }
                          frame True {
                            n186 = local read "Error Message"() -> (w422:string)
                            n187 = One Button Dialog(message=w422) -> ()  [unwired: 1 in, 1 out]
                          }
                        }
                        n188 = local write "System Confirm Not Clicked"(w416) -> ()
                        n189 = local write "Setup Confirm"(w415) -> ()
                      }
                    }
                  }
                }
              }
            }
            n190 = local read "Stop"() -> (w201:bool)
            n191 = Or(x=w202, y=w201) -> (x .or. y?=w200:bool)
            n192 = disable-structure shown="Disabled" {
              disable-tunnel: 400 -> [w208 _]
              frame Disabled {
                n193 = event shown="[1]" {
                  selector: _ -> [_ _]
                  dyn-events: _ -> [_ _]
                  timeout: w208 -> [_ _]
                  event Timeout {
                    n194 = event-data() -> ()  [unwired: 1 in, 3 out]
                  }
                  event #1 (no event record) {
                    n195 = event-data() -> ()  [unwired: 1 in, 6 out]
                    n196 = local read "Setup Confirm"() -> (w209:bool)
                    n197 = local read "Reaction Scheme Confirm"() -> (w210:bool)
                    n198 = Not(x=w209) -> (.not. x?=w212:bool)
                    n199 = And(x=w210, y=w212) -> (x .and. y?=w211:bool)
                    n200 = case shown="True" w211 {
                      frame False {
                      }
                      frame True {
                        w214 = u16 0 items=["                     Bypass", "                Hot Reactor", "                 Separator"] ("BAY 5")
                        w215 = u16 0 items=["                     Bypass", "                Hot Reactor", "                  Separator"] ("BAY 4")
                        w216 = u16 0 items=["                     Bypass", "                 Hot Reactor", "                  Separator"] ("BAY 3")
                        w217 = u16 0 items=["                     Bypass", "                Hot Reactor", "                  Separator"] ("BAY 2")
                        w218 = u16 0 items=["                 Bypass", "             Hot Reactor", "               Separator"] ("BAY 1")
                        n201 = local write "BAY 3"(w216) -> ()
                        n202 = local write "BAY 4"(w215) -> ()
                        n203 = local write "BAY 5"(w214) -> ()
                        n204 = local write "BAY 2"(w217) -> ()
                        n205 = local write "BAY 1"(w218) -> ()
                        n206 = local write "Synthesis Route Array"(string[][] [["3-Br-Pyridine _ Biphenyl", "K2CO3", "PhB(OH)2", "", "", ""]] ("Synthesis Route Array")) -> ()
                      }
                    }
                  }
                }
              }
              frame Enabled {
              }
            }
            n207 = disable-structure shown="Disabled" {
              disable-tunnel: 400 -> [w204 _]
              frame Disabled {
                n208 = event shown="[1]" {
                  selector: _ -> [_ _]
                  dyn-events: _ -> [_ _]
                  timeout: w204 -> [_ _]
                  event Timeout {
                    n209 = event-data() -> ()  [unwired: 1 in, 3 out]
                  }
                  event #1 (no event record) {
                    n210 = event-data() -> ()  [unwired: 1 in, 6 out]
                    n211 = call "File Dialog"("prompt"="Load previously saved xml file") -> ("selected path"=w206:path)  [unwired: 11 in, 3 out]
                    n212 = Path To String(path=w206) -> (string=w205:string)
                    n213 = script code="xmlDoc = xmlread(file_path);\nroot = xmlDoc.getDocumentElement();\nb = root.getChildNodes;\nrecipe = b.getElementsByTagName('Bay1').item(0);"("file_path"=w205) -> ()  [unwired: 1 in, 1 out]
                  }
                }
              }
              frame Enabled {
              }
            }
          }
        }
        frame #1 {
          n214 = local read "Stop"() -> (w424:bool)
          n215 = Not(x=w424) -> (.not. x?=w423:bool)
          n216 = case shown="True" w423 {
            tunnel: w425 -> [_ w428]
            frame False {
              "stop_button clicked" <- TRUE ("stop_button clicked")
            }
            frame True {
              # "Parameters Initilization"
              n217 = flat-sequence {
                tunnel: w428 -> [w430]
                tunnel: [w429] -> w427
                tunnel: w427 -> [w589]
                frame #0 {
                  # "Setup bays(RFID - verify)"
                  n218 = disable-structure shown="Disabled" {
                    frame Disabled {
                      n219 = local read "BAY 1"() -> ()  [unwired: 1 out]
                      n220 = local read "BAY 2"() -> ()  [unwired: 1 out]
                      n221 = local read "BAY 3"() -> ()  [unwired: 1 out]
                      n222 = local read "BAY 4"() -> ()  [unwired: 1 out]
                      n223 = local read "BAY 5"() -> ()  [unwired: 1 out]
                    }
                    frame Enabled {
                    }
                  }
                }
                frame #1 {
                  n224 = while {
                    tunnel: w430 -> [w433]
                    tunnel: [w432] -> w429
                    stop <- w436 stop-if-true
                    n225 = flat-sequence {
                      tunnel: [w450] -> w432
                      tunnel: w433 -> [w531]
                      tunnel: [w449] -> w431
                      frame #0 {
                        n226 = while {
                          stop <- w440 stop-if-true
                          n227 = event shown="[1] \"System Parameters Confirm Button\": Value Change" {
                            selector: _ -> [_ _]
                            dyn-events: _ -> [_ _]
                            timeout: u32 200 ("milliseconds to wait") -> [_ _]
                            tunnel: [FALSE TRUE] -> w438
                            event Timeout {
                              n228 = event-data() -> ()  [unwired: 1 in, 3 out]
                            }
                            event "System Parameters Confirm Button": Value Change {
                              n229 = event-data() -> ()  [unwired: 1 in, 5 out]
                              n230 = local write "System Parameters Confirm Button"(FALSE) -> ()
                            }
                          }
                          n231 = Wait (ms)(milliseconds to wait=u32 500) -> ()  [unwired: 1 out]
                          n232 = local read "Stop"() -> (w441:bool)
                          n233 = Or(x=w441, y=w438) -> (x .or. y?=w440:bool)
                        }
                      }
                      frame #1 {
                        w470 = 0 ("disabled index (col)")
                        w482 = 1 ("disabled index (col)")
                        # "Do while parameters have not been correctly entered"
                        n234 = local read "Bay Parameters"() -> (w469:T2)
                        n235 = local read "Synthesis Route Array"() -> (w483:string[][])
                        n236 = local read "Total Number of Experiments"() -> (w502:dbl)
                        n237 = Unbundle By Name(w469) -> ("Continue from previous optimization?"=w530:bool)
                        n238 = Unbundle By Name(w469) -> ("Excel File Name"=w532:string)
                        n239 = Unbundle By Name(w469) -> ("Matlab File"=w528:string)
                        n240 = Unbundle By Name(w469) -> ("Bay 1.Run at set flowrate"=w574:bool)
                        n241 = Unbundle By Name(w469) -> ("Bay 1.Pump 1 Flowrate"=w580:dbl)
                        n242 = Unbundle By Name(w469) -> ("Bay 1.Pump 2 Flowrate"=w579:dbl)
                        n243 = Unbundle By Name(w469) -> ("Bay 2.Run at set flowrate"=w572:bool)
                        n244 = Unbundle By Name(w469) -> ("Bay 2.Pump 3 Flowrate"=w578:dbl)
                        n245 = Unbundle By Name(w469) -> ("Bay 3.Pump 4 Flowrate"=w577:dbl)
                        n246 = Unbundle By Name(w469) -> ("Bay 3.Run at set flowrate"=w571:bool)
                        n247 = Unbundle By Name(w469) -> ("Bay 4.Run at set flowrate"=w568:bool)
                        n248 = Unbundle By Name(w469) -> ("Bay 4.Pump 5 Flowrate"=w576:dbl)
                        n249 = Unbundle By Name(w469) -> ("Bay 5.Pump 6 Flowrate"=w575:dbl)
                        n250 = Unbundle By Name(w469) -> ("Bay 5.Run at set flowrate"=w567:bool)
                        n251 = Index Array(array=w483, index (row)=3, index (col)=w482) -> (element=w476:string)
                        n252 = Index Array(array=w483, index (row)=2, index (col)=w482) -> (element=w474:string)
                        n253 = Index Array(array=w483, index (row)=1, index (col)=w482) -> (element=w472:string)
                        n254 = Index Array(array=w483, index (row)=0, index (col)=w482) -> (element=w485:string)
                        n255 = Index Array(array=w483, index (row)=4, index (col)=w482) -> (element=w478:string)
                        n256 = Index Array(array=w483, index (row)=5, index (col)=w482) -> (element=w480:string)
                        n257 = Build Array(w485, w472, w474, w476, w478, w480) -> (w486:string[])
                        n258 = Index Array(array=w483, index (row)=0 ("index"), index (col)=w470) -> (element=w508:string)
                        n259 = for {
                          tunnel: w486 -> [w582] mode=indexing
                          tunnel: [w581] -> w471 mode=indexing
                          n260 = script code="ctemp1 = str2num(c_temp);"("c_temp"=w582) -> ("ctemp1"=w581:dbl)  [unwired: 1 in, 1 out]
                        }
                        n261 = Boolean To (0,1)(Boolean=w572) -> (0, 1=w527:i16)
                        n262 = Boolean To (0,1)(Boolean=w568) -> (0, 1=w569:i16)
                        n263 = Boolean To (0,1)(Boolean=w571) -> (0, 1=w570:i16)
                        n264 = Boolean To (0,1)(Boolean=w530) -> (0, 1=w529:i16)
                        n265 = Boolean To (0,1)(Boolean=w574) -> (0, 1=w573:i16)
                        n266 = Boolean To (0,1)(Boolean=w567) -> (0, 1=w566:i16)
                        n267 = Index Array(array=w483, index (row)=1 ("index"), index (col)=w470) -> (element=w503:string)
                        n268 = Index Array(array=w483, index (row)=2 ("index"), index (col)=w470) -> (element=w504:string)
                        n269 = Unbundle By Name(w469) -> ("Bay 1.optimize_temp"=w565:bool)
                        n270 = Unbundle By Name(w469) -> ("Bay 1.optimize_tau"=w563:bool)
                        n271 = Unbundle By Name(w469) -> ("Bay 2.optimize_temp"=w561:bool)
                        n272 = Unbundle By Name(w469) -> ("Bay 2.optimize_tau"=w559:bool)
                        n273 = Unbundle By Name(w469) -> ("Bay 3.optimize_temp"=w557:bool)
                        n274 = Unbundle By Name(w469) -> ("Bay 3.optimize_tau"=w555:bool)
                        n275 = Unbundle By Name(w469) -> ("Bay 4.optimize_temp"=w553:bool)
                        n276 = Unbundle By Name(w469) -> ("Bay 4.optimize_tau"=w551:bool)
                        n277 = Index Array(array=w483, index (row)=3 ("index"), index (col)=w470) -> (element=w505:string)
                        n278 = Boolean To (0,1)(Boolean=w553) -> (0, 1=w552:i16)
                        n279 = Boolean To (0,1)(Boolean=w551) -> (0, 1=w550:i16)
                        n280 = Index Array(array=w483, index (row)=4 ("index"), index (col)=w470) -> (element=w506:string)
                        n281 = Boolean To (0,1)(Boolean=w555) -> (0, 1=w554:i16)
                        n282 = Boolean To (0,1)(Boolean=w561) -> (0, 1=w560:i16)
                        n283 = Boolean To (0,1)(Boolean=w565) -> (0, 1=w564:i16)
                        n284 = Boolean To (0,1)(Boolean=w559) -> (0, 1=w558:i16)
                        n285 = Boolean To (0,1)(Boolean=w563) -> (0, 1=w562:i16)
                        n286 = Boolean To (0,1)(Boolean=w557) -> (0, 1=w556:i16)
                        n287 = Unbundle By Name(w469) -> ("Bay 5.optimize_temp"=w549:bool)
                        n288 = Unbundle By Name(w469) -> ("Bay 5.optimize_tau"=w547:bool)
                        n289 = Index Array(array=w483, index (row)=5 ("index"), index (col)=w470) -> (element=w507:string)
                        n290 = Boolean To (0,1)(Boolean=w549) -> (0, 1=w548:i16)
                        n291 = Boolean To (0,1)(Boolean=w547) -> (0, 1=w546:i16)
                        n292 = Build Array(w564, w562, w560, w558, w556, w554, w552, w550, w548, w546) -> (w545:i16[])
                        n293 = Unbundle By Name(w469) -> ("Bay 1.Temperature Params"=w542:dbl[])
                        n294 = Unbundle By Name(w469) -> ("Bay 2.Temperature Params"=w541:dbl[])
                        n295 = Unbundle By Name(w469) -> ("Bay 2.Resisdence time params"=w536:dbl[])
                        n296 = Unbundle By Name(w469) -> ("Bay 3.Temperature Params"=w540:dbl[])
                        n297 = Unbundle By Name(w469) -> ("Bay 3.Resisdence time params"=w535:dbl[])
                        n298 = Unbundle By Name(w469) -> ("Bay 4.Temperature Params"=w539:dbl[])
                        n299 = Unbundle By Name(w469) -> ("Bay 4.Resisdence time params"=w534:dbl[])
                        n300 = Unbundle By Name(w469) -> ("Bay 5.Temperature Params"=w538:dbl[])
                        n301 = Unbundle By Name(w469) -> ("Bay 5.Resisdence time params"=w533:dbl[])
                        n302 = Unbundle By Name(w469) -> ("Bay 1.pump params 2"=w501:dbl[])
                        n303 = Unbundle By Name(w469) -> ("Bay 1.pump params 1"=w537:dbl[])
                        n304 = Unbundle By Name(w469) -> ("Bay 1.Run at set temperature"=w492:bool)
                        n305 = Unbundle By Name(w469) -> ("Bay 2.Run at set temperature"=w490:bool)
                        n306 = Unbundle By Name(w469) -> ("Bay 3.Run at set temperature"=w489:bool)
                        n307 = Unbundle By Name(w469) -> ("Bay 4.Run at set temperature"=w488:bool)
                        n308 = Unbundle By Name(w469) -> ("Bay 5.Run at set temperature"=w487:bool)
                        n309 = Unbundle By Name(w469) -> ("Bay 3.Temperature"=w498:dbl)
                        n310 = Unbundle By Name(w469) -> ("Bay 1.Temperature"=w500:dbl)
                        n311 = Unbundle By Name(w469) -> ("Bay 2.Temperature"=w499:dbl)
                        n312 = Unbundle By Name(w469) -> ("Bay 4.Temperature"=w497:dbl)
                        n313 = Unbundle By Name(w469) -> ("Bay 5.Temperature"=w496:dbl)
                        n314 = Unbundle By Name(w469) -> ("Bay 3.pump_num_ratio"=w521:dbl)
                        n315 = Unbundle By Name(w469) -> ("Bay 4.pump_num_ratio"=w518:dbl)
                        n316 = Unbundle By Name(w469) -> ("Bay 5.pump_num_ratio"=w515:dbl)
                        n317 = Unbundle By Name(w469) -> ("Bay 2.pump_num_ratio"=w524:dbl)
                        n318 = Unbundle By Name(w469) -> ("Bay 4.pump_at_ratio"=w520:bool)
                        n319 = Boolean To (0,1)(Boolean=w520) -> (0, 1=w519:i16)
                        n320 = Unbundle By Name(w469) -> ("Bay 3.pump_at_ratio"=w523:bool)
                        n321 = Boolean To (0,1)(Boolean=w523) -> (0, 1=w522:i16)
                        n322 = Unbundle By Name(w469) -> ("Bay 5.pump_at_ratio"=w517:bool)
                        n323 = Boolean To (0,1)(Boolean=w517) -> (0, 1=w516:i16)
                        n324 = Unbundle By Name(w469) -> ("Bay 2.pump_at_ratio"=w526:bool)
                        n325 = Boolean To (0,1)(Boolean=w526) -> (0, 1=w525:i16)
                        n326 = Build Array(w500, w499, w498, w497, w496) -> (w495:dbl[])
                        n327 = Build Array(w492, w490, w489, w488, w487) -> (w491:bool[])
                        n328 = local read "Syringe_pump?"() -> (w448:bool)
                        n329 = for {
                          N: 5 -> [_]
                          tunnel: w491 -> [w586] mode=indexing
                          tunnel: [w585] -> w493 mode=indexing
                          n330 = Select(t=1.0, s=w586, f=0.0) -> (s? t:f=w585:dbl)
                        }
                        n331 = Unbundle By Name(w469) -> ("Internal Standard?"=w460:bool)
                        n332 = Unbundle By Name(w469) -> ("increas_decrease_hplc_peak"=w461:bool)
                        n333 = Unbundle By Name(w469) -> ("Hplc Wait time(min)"=w453:dbl)
                        n334 = Unbundle By Name(w469) -> ("Total Number of Experiments 2"=w452:dbl)
                        n335 = Unbundle By Name(w469) -> ("hplc_start"=w457:dbl)
                        n336 = Unbundle By Name(w469) -> ("ISTD start"=w455:dbl)
                        n337 = Unbundle By Name(w469) -> ("hplc_end"=w456:dbl)
                        n338 = Unbundle By Name(w469) -> ("throughput_yield"=w462:bool)
                        n339 = Unbundle By Name(w469) -> ("ISTD end"=w454:dbl)
                        n340 = Select(t=1.0, s=w448, f=0.0) -> (s? t:f=w447:dbl)
                        n341 = Select(t=1.0, s=w461, f=0.0) -> (s? t:f=w459:dbl)
                        n342 = Select(t=1.0, s=w460, f=0.0) -> (s? t:f=w458:dbl)
                        n343 = Select(t=0.0, s=w462, f=1.0) -> (s? t:f=w451:dbl)
                        n344 = script code="system_error = 0;\nnumPeaks = 1;\nstart_phase_time = 1;\nis_redo_exp = 0;\nFvalues = [];\nHPLC_Area = [];\n\nT1_span = [1 1]; T2_span = [1 1]; T3_span = [1 1]; T4_span = [1 1]; T5_span = [1 1];\nT_span = [T1_span;T2_span;T3_span;T4_span;T5_span];\n p1_span =  [1 1]; p2_span =  [1 1]; p3_span =  [1 1]; p4_span =  [1 1]; p5_span =  [1 1];  p6_span =  [1 1];\nOpt_params = [0 0 0 0 0 0 0 0 0 0 0];\nT_params = [T1_params;T2_params;T3_params;T4_params;T5_params];\npump_params = [pump1_params;pump2_params;pump3_params;pump4_params;pump5_params;pump6_params];\nopt_ctr = 0;ncall = 100;record_data = true;\nT1_SP = 23; T2_SP = 23; T3_SP = 23; T4_SP = 23; T5_SP = 23;\nT_span = [T1_span;T2_span;T3_span;T4_span;T5_span];\np_span = [p1_span;p2_span;p3_span;p4_span;p5_span;p6_span];\nno_errors = 1;\nP1 = 0; P2 =0; P3 = 0; P4 = 0; P5 = 0; P6 = 0;\nP = [P1, P2, P3,P4, P5, P6];\nis_first_set_of_exp = true;\nerror_message = 'System has no errors to report';\naddpath(genpath('C:\\Users\\HPLC\\Dropbox (MIT)\\MoD Files\\MATLAB'))\n%addpath(genpath('C:\\Users\\Admin\\Dropbox (MIT)\\MoD Files\\MATLAB'))\nallMSData = [];allHPLCData = [];allHPLCFile = [];\nBay_ratio = [0,Bay2_ratio,Bay3_ratio,Bay4_ratio,Bay5_ratio];\nBay_pump_ratio = [1, Bay2_pump_ratio, Bay3_pump_ratio, Bay4_pump_ratio, Bay5_pump_ratio];\nP_setrate = [P1_setrate, P2_setrate, P3_setrate, P4_setrate, P5_setrate, P6_setrate];\nuse_flowrate = [use_flowrate1, use_flowrate2,use_flowrate3, use_flowrate4, use_flowrate5];\npump_chem_name= []\nCurrExp = 1;\n% ****************************************************************************************************\n%Setup optimization\n   setup_optimization_params;\n   initialize_opt = 0;\n   nstop0 = 0;\n%*****************************************************************************************************\n% Setup excel and xml file writing\npath(path, pa);\nnumMSSig = 1;\nsetup_excel_output;\n%***************************************************************************************************\nredo = false;\nncall = ncall_in;"("use_flowrate1"=w573, "P1_setrate"=w580, "P2_setrate"=w579, "P3_setrate"=w578, "P4_setrate"=w577, "P5_setrate"=w576, "P6_setrate"=w575, "use_flowrate2"=w527, "use_flowrate3"=w570, "use_flowrate4"=w569, "use_flowrate5"=w566, "Optimize_params"=w545, "T1_params"=w542, "T2_params"=w541, "T3_params"=w540, "T4_params"=w539, "T5_params"=w538, "pump1_params"=w537, "pump3_params"=w536, "pump4_params"=w535, "pump5_params"=w534, "pump6_params"=w533, "xl_file"=w532, "pa"=w531, "Continue"=w529, "matlabsavefile"=w528, "Bay2_ratio"=w525, "Bay2_pump_ratio"=w524, "Bay3_ratio"=w522, "Bay3_pump_ratio"=w521, "Bay4_ratio"=w519, "Bay4_pump_ratio"=w518, "Bay5_ratio"=w516, "Bay5_pump_ratio"=w515, "pump1_chem"=w508, "pump6_chem"=w507, "pump5_chem"=w506, "pump4_chem"=w505, "pump3_chem"=w504, "pump2_chem"=w503, "Pump_concen"=w471, "ncall_in"=w502, "pump2_params"=w501, "T_SP"=w495, "Run_at_T_SP"=w493, "dcr_hplc_peak"=w459, "use_internal_std"=w458, "hplc_peak_start"=w457, "hplc_peak_end"=w456, "ISTD_start"=w455, "ISTD_end"=w454, "hplc_wait_time"=w453, "tot_num_exp"=w452, "throughput_yield"=w451, "syringe_pump"=w447) -> ("no_errors"=w544:dbl, "error_message"=w543:string)  [unwired: 1 in, 1 out]
                        n345 = Not Equal To 0?(x=w544) -> (x != 0?=w449:bool)
                        n346 = Not(x=w449) -> (.not. x?=w450:bool)
                        n347 = case shown="False" w450 {
                          tunnel: w543 -> [_ w588]
                          frame False {
                            n348 = local write "Setup Confirm 2"(TRUE ("Setup Confirm 2")) -> ()
                          }
                          frame True {
                            n349 = One Button Dialog(message=w588) -> ()  [unwired: 1 in, 1 out]
                          }
                        }
                      }
                    }
                    n350 = local read "Stop"() -> (w435:bool)
                    n351 = Or(x=w431, y=w435) -> (x .or. y?=w436:bool)
                    n352 = Wait (ms)(milliseconds to wait=u32 500) -> ()  [unwired: 1 out]
                  }
                }
                frame #2 {
                  n353 = local write "System Error"(w589) -> ()
                }
              }
            }
          }
        }
        frame #2 {
          # "Run Initial diagnostics"
        }
        frame #3 {
          # "Run System"
          n354 = while {
            tunnel: w590 -> [w1324]
            stop <- w1328 stop-if-true
            n355 = local read "running?"() -> (w1323:bool)
            n356 = local read "Temperature Control 1"() -> (w1325:bool)
            n357 = And(x=w1323, y=w1325) -> (x .and. y?=w1326:bool)
            n358 = case shown="True" w1326 {
              tunnel: w1324 -> [_ w1330]
              frame False {
                n359 = local write "Temp SS? 1"(TRUE ("Temp SS? 1")) -> ()
              }
              frame True {
                # "Bay 1 Temperature Controller"
                n360 = local read "Temperature SP 1"() -> (w1331:dbl)
                n361 = local read "Temperature 1"() -> (w1335:dbl)
                n362 = local read "SSR Duration 1"() -> (w1350:dbl)
                n363 = call-poly <vilib>:"PID Online Autotuning.vi"("setpoint"=w1331, "manipulated variable"=w1350, "autotuning parameters"=T9 {"type of controller"=enum."PID", "relay cycles"=3, "relay amplitude"=1.0, "control specifications"=enum."Normal", "PV noise level"=0.1} ("Autotuning Parameters R1"), "process variable"=w1335, "PID gains in"=T8 {"Proportional gain Kc"=0.38538, "Integral time Ti (sec)"=0.524375, "Derivative time Ti (sec)"=0.12585} ("PID gains 2")) -> ("setpoint out"=w1356:dbl, "process variable out"=w1355:dbl, "PID gains out"=w1352:T17)  [unwired: 6 in, 2 out]
                n364 = call <vilib>:"PID Autotuning (Temperature).vi"("desired temperature"=w1356, "measured temperature"=w1355, "plant parameters in"=w1352, "output range"=cluster{"output high":dbl, "output low":dbl} {"output high"=3.0, "output low"=-1.0} ("Output range")) -> ("output"=w1348:dbl)  [unwired: 12 in, 3 out]
                n365 = local write "SSR Duration 1"(w1348) -> ()
                n366 = Subtract(x=w1331, y=w1335) -> (x-y=w1342:dbl)
                n367 = Absolute Value(x=w1342) -> (abs(x)=w1345:dbl)
                n368 = Multiply(x=1000.0, y=w1348) -> (x*y=w1346:dbl)
                n369 = Greater Than 0?(x=w1346) -> (x > 0?=w1340:bool)
                n370 = Less Or Equal?(x=w1345, y=1.2) -> (x <= y?=w1343:bool)
                n371 = Greater?(x=w1331, y=w1335) -> (0:w1341:bool)
                n372 = And(x=w1340, y=w1341) -> (x .and. y?=w1338:bool)
                n373 = local write "Temp SS? 1"(w1343) -> ()
                n374 = Subtract(x=w1335, y=10.0) -> (x-y=w1336:dbl)
                n375 = Less?(x=w1336, y=w1331) -> (x < y?=w1339:bool)
                n376 = And(x=w1339, y=w1338) -> (x .and. y?=w1337:bool)
                n377 = case shown="True" w1337 {
                  tunnel: [errorcluster {"status"=FALSE, "code"=0, "source"=""} ("error out") w1366] -> _
                  tunnel: 2 -> [_ w1363]
                  tunnel: w1346 -> [w1360 w1364]
                  tunnel: [0.0 w1368] -> w1333
                  tunnel: w1331 -> [_ w1367]
                  tunnel: w1330 -> [_ w1365]
                  frame False {
                    n378 = Absolute Value(x=w1360) -> (abs(x)=w1361:dbl)
                    n379 = Wait (ms)(milliseconds to wait=w1361) -> ()  [unwired: 1 out]
                  }
                  frame True {
                    n380 = call "TurnOnRelayArduino.vi"("channel"=w1363, "duration"=w1364, "LINX Resource"=w1365) -> ("error out"=w1366:errorcluster)  [unwired: 7 in, 1 out]
                    n381 = script code="tempdiff1= SP1 - T1;\nif tempdiff1 > 10\n  if slope1 < .01\n     temp_check1 = temp_check1 + 1;\n  else\n      temp_check1 =0;\n  end\nend\n\nif temp_check1 > 9\n  temp_error1 = 1\nend"("SP1"=w1367) -> ("temp_error1"=w1368:dbl)  [unwired: 1 in, 1 out]
                  }
                }
                n382 = Not Equal To 0?(x=w1333) -> (x != 0?=w1332:bool)
                n383 = case shown="True" w1332 {
                  frame False {
                  }
                  frame True {
                    n384 = local write "Error Message"("Bay 1 Temperature Heating Error") -> ()
                  }
                }
                n385 = case shown="True" w1332 {
                  tunnel: w1332 -> [_ w1358]
                  frame False {
                  }
                  frame True {
                    n386 = local write "System Error"(w1358) -> ()
                    n387 = local write "Stop"(w1358) -> ()
                  }
                }
              }
            }
            n388 = Wait (ms)(milliseconds to wait=u32 400) -> ()  [unwired: 1 out]
            n389 = local read "Stop"() -> (w1328:bool)
          }
          n390 = local read "Bay Parameters"() -> (w594:T2)
          n391 = while {
            tunnel: w590 -> [w1278]
            stop <- w1282 stop-if-true
            n392 = local read "running?"() -> (w1277:bool)
            n393 = local read "Temperature Control 2"() -> (w1279:bool)
            n394 = And(x=w1277, y=w1279) -> (x .and. y?=w1280:bool)
            n395 = case shown="True" w1280 {
              tunnel: w1278 -> [_ w1284]
              frame False {
                n396 = local write "Temp SS? 2"(TRUE ("Temp SS? 2")) -> ()
              }
              frame True {
                # "Bay 2 Temperature Controller"
                n397 = local read "Temperature SP 2"() -> (w1286:dbl)
                n398 = local read "Temperature 2"() -> (w1289:dbl)
                n399 = local read "SSR Duration 2"() -> (w1307:dbl)
                n400 = call-poly <vilib>:"PID Online Autotuning.vi"("setpoint"=w1286, "manipulated variable"=w1307, "autotuning parameters"=T9 {"type of controller"=enum."PID", "relay cycles"=3, "relay amplitude"=1.0, "control specifications"=enum."Normal", "PV noise level"=0.1} ("Autotuning Parameters R1"), "process variable"=w1289, "PID gains in"=T8 {"Proportional gain Kc"=0.38538, "Integral time Ti (sec)"=0.524375, "Derivative time Ti (sec)"=0.12585} ("PID gains 2")) -> ("setpoint out"=w1305:dbl, "process variable out"=w1304:dbl, "PID gains out"=w1310:T17)  [unwired: 6 in, 2 out]
                n401 = call <vilib>:"PID Autotuning (Temperature).vi"("desired temperature"=w1305, "measured temperature"=w1304, "plant parameters in"=w1310, "output range"=cluster{"output high":dbl, "output low":dbl} {"output high"=3.0, "output low"=-1.0} ("Output range")) -> ("output"=w1300:dbl)  [unwired: 12 in, 3 out]
                n402 = local write "SSR Duration 2"(w1300) -> ()
                n403 = Greater?(x=w1286, y=w1289) -> (0:w1295:bool)
                n404 = Multiply(x=1000.0, y=w1300) -> (x*y=w1302:dbl)
                n405 = Greater Than 0?(x=w1302) -> (x > 0?=w1294:bool)
                n406 = And(x=w1294, y=w1295) -> (x .and. y?=w1292:bool)
                n407 = Subtract(x=w1286, y=w1289) -> (x-y=w1297:dbl)
                n408 = Absolute Value(x=w1297) -> (abs(x)=w1299:dbl)
                n409 = Subtract(x=w1289, y=10.0) -> (x-y=w1291:dbl)
                n410 = Less Or Equal?(x=w1299, y=1.2) -> (x <= y?=w1296:bool)
                n411 = local write "Temp SS? 2"(w1296) -> ()
                n412 = Less?(x=w1291, y=w1286) -> (x < y?=w1293:bool)
                n413 = And(x=w1293, y=w1292) -> (x .and. y?=w1288:bool)
                n414 = case shown="True" w1288 {
                  tunnel: [errorcluster {"status"=FALSE, "code"=0, "source"=""} ("error out") w1320] -> _
                  tunnel: 3 -> [_ w1317]
                  tunnel: w1302 -> [w1314 w1318]
                  tunnel: [0.0 w1322] -> w1287
                  tunnel: w1286 -> [_ w1321]
                  tunnel: w1284 -> [_ w1319]
                  frame False {
                    n415 = Absolute Value(x=w1314) -> (abs(x)=w1315:dbl)
                    n416 = Wait (ms)(milliseconds to wait=w1315) -> ()  [unwired: 1 out]
                  }
                  frame True {
                    n417 = call "TurnOnRelayArduino.vi"("channel"=w1317, "duration"=w1318, "LINX Resource"=w1319) -> ("error out"=w1320:errorcluster)  [unwired: 7 in, 1 out]
                    n418 = script code="tempdiff2= SP2 - T2;\nif tempdiff2 > 10\n  if slope2 < .01\n     temp_check2 = temp_check2 + 1;\n  else\n      temp_check2 =0;\n  end\nend\n\nif temp_check2 > 9\n  temp_error2 = 1\nend"("SP2"=w1321) -> ("temp_error2"=w1322:dbl)  [unwired: 1 in, 1 out]
                  }
                }
                n419 = Not Equal To 0?(x=w1287) -> (x != 0?=w1285:bool)
                n420 = case shown="True" w1285 {
                  frame False {
                  }
                  frame True {
                    n421 = local write "Error Message"("Bay 2 Temperature Heating Error") -> ()
                  }
                }
                n422 = case shown="True" w1285 {
                  tunnel: w1285 -> [_ w1312]
                  frame False {
                  }
                  frame True {
                    n423 = local write "Stop"(w1312) -> ()
                    n424 = local write "System Error"(w1312) -> ()
                  }
                }
              }
            }
            n425 = local read "Stop"() -> (w1282:bool)
            n426 = Wait (ms)(milliseconds to wait=u32 400) -> ()  [unwired: 1 out]
          }
          n427 = local read "Stop"() -> (w591:bool)
          n428 = Not(x=w591) -> (.not. x?=w593:bool)
          n429 = case shown="True" w593 {
            tunnel: w594 -> [_ w599]
            tunnel: w592 -> [_ w598]
            tunnel: w590 -> [_ w597]
            frame False {
            }
            frame True {
              n430 = while {
                tunnel: w599 -> [w613]
                tunnel: w598 -> [w605]
                tunnel: w597 -> [w600]
                i -> [w612]
                stop <- w606 stop-if-true
                n431 = local read "running?"() -> (w601:bool)
                n432 = Wait (ms)(milliseconds to wait=u32 1000) -> ()  [unwired: 1 out]
                n433 = Increment(x=w612) -> (x+1=w602:i32)
                n434 = case shown="True" w601 {
                  tunnel: w612 -> [w618 _]
                  tunnel: w613 -> [_ _]
                  tunnel: [w620 w624] -> w603
                  tunnel: [0.0 w625] -> w608
                  tunnel: w605 -> [_ w623]
                  tunnel: w600 -> [_ w621]
                  frame False {
                    # "STANDBY MODE"
                    n435 = Add(x=w618, y=2.0) -> (x+y=w620:dbl)
                  }
                  frame True {
                    n436 = flat-sequence {
                      tunnel: w623 -> [w627]
                      tunnel: [w627] -> w622
                      tunnel: [w637] -> w625
                      tunnel: [200.0] -> w624
                      tunnel: w622 -> [w635]
                      tunnel: w621 -> [w629]
                      frame #0 {
                        n437 = local write "stop_xl_write"(FALSE ("stop_xl_write")) -> ()
                      }
                      frame #1 {
                        # "Increase flowrate of dilution stream"
                        # "Wait mixed stream reaches SL"
                        # "SNOBFIT"
                        # "Optimize"
                        # "Run Experimental Conditions"
                        # "Optimize/Synthesize"
                        n438 = local read "Syringe_pump?"() -> (w628:bool)
                        n439 = local read "Stop"() -> (w632:bool)
                        n440 = Not(x=w632) -> (.not. x?=w631:bool)
                        n441 = case shown="True" w631 {
                          tunnel: [1.0 w660] -> w640
                          tunnel: [w648 w659] -> w634
                          tunnel: [0.0 w658] -> w633
                          tunnel: [w648 w657] -> w630
                          tunnel: w628 -> [_ w654]
                          frame False {
                            w648 = dbl[] []
                          }
                          frame True {
                            n442 = Select(t=1.0, s=w654, f=0.0) -> (s? t:f=w653:dbl)
                            n443 = script code="optimization_main_loop"("syringe_pump"=w653) -> ("Conditions_Array"=w659:dbl[], "opt_ctr"=w660:dbl, "P_tot"=w658:dbl, "tau_array"=w657:dbl[], "experiment_history"=w655:dbl[][])  [unwired: 1 in, 1 out]
                            n444 = call-poly <vilib>:"Array To Matrix.vi"("Real 2D Array"=w655) -> ("Real Matrix"=w656:T18)
                            n445 = local write "experiment history"(w656) -> ()
                          }
                        }
                        "P_tot" <- w633
                        n446 = local read "COMM Port :: Milligat Pumps"() -> (w641:refnum<visa-resource-name>)
                        n447 = Equal?(x=w640, y=1.0) -> (x = y?=w638:bool)
                        n448 = flat-sequence {
                          tunnel: w634 -> [w1122]
                          tunnel: w630 -> [w1116]
                          frame #0 {
                            # "Start recording data"
                            n449 = Index Array(array=w1122, index=5) -> (element=w1134:dbl)
                            n450 = Index Array(array=w1122, index=0) -> (element=w1129:dbl)
                            n451 = Index Array(array=w1122, index=1) -> (element=w1130:dbl)
                            n452 = Index Array(array=w1122, index=2) -> (element=w1132:dbl)
                            n453 = Index Array(array=w1122, index=3) -> (element=w1131:dbl)
                            n454 = Index Array(array=w1122, index=4) -> (element=w1133:dbl)
                            n455 = local write "Pump setpoint(ul/min) 2"(w1130) -> ()
                            n456 = local write "Pump setpoint(ul/min) 4"(w1132) -> ()
                            n457 = local write "Pump setpoint(ul/min) 5"(w1133) -> ()
                            n458 = local write "Pump setpoint(ul/min) 3"(w1131) -> ()
                            n459 = local write "Pump setpoint(ul/min) 6"(w1134) -> ()
                            n460 = local write "Pump setpoint(ul/min) 1"(w1129) -> ()
                            n461 = Index Array(array=w1116, index=0) -> (element=w1121:dbl)
                            n462 = Index Array(array=w1116, index=4) -> (element=w1120:dbl)
                            n463 = Index Array(array=w1116, index=3) -> (element=w1119:dbl)
                            n464 = Index Array(array=w1116, index=2) -> (element=w1118:dbl)
                            n465 = Index Array(array=w1116, index=1) -> (element=w1117:dbl)
                            n466 = local write "tau 2"(w1117) -> ()
                            n467 = local write "tau 3"(w1118) -> ()
                            n468 = local write "tau 4"(w1119) -> ()
                            n469 = local write "tau 5"(w1120) -> ()
                            n470 = local write "tau 1"(w1121) -> ()
                          }
                        }
                        n471 = flat-sequence {
                          tunnel: w641 -> [w664]
                          tunnel: w634 -> [w663]
                          tunnel: w638 -> [w662]
                          tunnel: [w662] -> w647
                          tunnel: w635 -> [w661]
                          tunnel: w647 -> [w830]
                          tunnel: [w830] -> w646
                          tunnel: w646 -> [w850]
                          tunnel: [w848] -> w645
                          tunnel: w634 -> [w874]
                          tunnel: w645 -> [w873]
                          tunnel: w629 -> [w872]
                          tunnel: [w1052] -> w644
                          tunnel: w644 -> [w1065]
                          tunnel: [w1065] -> w643
                          tunnel: w643 -> [w1073]
                          tunnel: [w1073] -> w642
                          tunnel: [w1110] -> w637
                          tunnel: w642 -> [w1110]
                          frame #0 {
                            # "Setup pump flowrates and temperature setpoints"
                            n472 = stacked-sequence {
                              tunnel: w664 -> [w690 _ _ _ _]
                              tunnel: w664 -> [_ w736 _ _ _]
                              tunnel: w664 -> [_ _ w764 _ _]
                              tunnel: w664 -> [_ _ _ w792 _]
                              tunnel: w664 -> [_ _ _ _ w820]
                              tunnel: w663 -> [w687 w734 w762 w790 w817]
                              tunnel: w662 -> [w679 w729 w757 w785 w813]
                              tunnel: w661 -> [w677 _ _ _ _]
                              frame #0 {
                                # "Bay 1"
                                n473 = local read "Syringe_pump?"() -> (w678:bool)
                                n474 = Index Array(array=w687, index=0) -> (element=w685:dbl)
                                n475 = local read "BAY 1"() -> (w672:u16)
                                n476 = Index Array(array=w687, index=1) -> (element=w684:dbl)
                                n477 = Index Array(array=w687, index=6) -> (element=w667:dbl)
                                n478 = script code="MATLAB script"("T1_SP"=w667) -> ()  [unwired: 1 in, 1 out]
                                n479 = Less Or Equal?(x=w672, y=u16 4) -> (x <= y?=w674:bool)
                                n480 = Greater Or Equal?(x=w672, y=u16 1) -> (x >= y?=w675:bool)
                                n481 = Not Equal?(x=23.0, y=w667) -> (x != y?=w668:bool)
                                n482 = And(x=w675, y=w674) -> (x .and. y?=w676:bool)
                                n483 = Greater Than 0?(x=w685) -> (x > 0?=w683:bool)
                                n484 = And(x=w683, y=w679) -> (x .and. y?=w682:bool)
                                n485 = Greater Than 0?(x=w684) -> (x > 0?=w681:bool)
                                n486 = Wait (ms)(milliseconds to wait=u32 300) -> ()  [unwired: 1 out]
                                n487 = And(x=w681, y=w679) -> (x .and. y?=w680:bool)
                                n488 = And(x=w676, y=w679) -> (x .and. y?=w666:bool)
                                n489 = And(x=w668, y=w666) -> (x .and. y?=w665:bool)
                                n490 = case shown="False" w678 {
                                tunnel: w690 -> [w693 _]
                                tunnel: w684 -> [w692 w700]
                                tunnel: w680 -> [w691 w701]
                                tunnel: w677 -> [_ w699]
                                frame False {
                                n491 = case shown="True" w691 {
                                tunnel: w693 -> [w695 w696]
                                tunnel: w692 -> [_ w697]
                                frame False {
                                n492 = call "PumpStop.vi"("Pump Address"="f", "Pump COMM Port"=w695) -> ()  [unwired: 9 in, 1 out]
                                }
                                frame True {
                                n493 = call "PumpDispense.vi"("Flowrate(ul/min)"=w697, "Pump Address"="f", "Pump COMM Port"=w696) -> ()  [unwired: 7 in, 2 out]
                                }
                                }
                                }
                                frame True {
                                n494 = case shown="False" w701 {
                                tunnel: w700 -> [_ w703]
                                tunnel: w699 -> [w702 w704]
                                frame False {
                                n495 = call <instrlib>:"Stop Pump.vi"("VISA resource name"=w702) -> ()  [unwired: 9 in, 2 out]
                                }
                                frame True {
                                w705 = u16 0 items=["Infuse", "Withdraw"] ("Run Direction (0:Infuse)")
                                w706 = u32 4 items=["milliliters per hour (ml/hr)", "milliliters per minute (ml/min)", "milliliters per second (ml/sec)", "microliters per hour (ul/hr)", "microliters per minute (ul/min)", "microliters per second (ul/sec)", "nanoliters per hour (nl/hr)", "nanoliters per minute (nl/min)", "nanoliters per second (nl/sec)", "picoliters per hour (pl/hr)", "picoliters per minute (pl/min)", "picoliters per second (pl/sec)"] ("Flow Rate Units (1:ml/min)")
                                w707 = u16 0 items=["Infuse", "Withdraw"] ("Pump Direction (0:Infuse)")
                                n496 = call <instrlib>:"Configure Flow Rate & Direction.vi"("VISA resource name"=w704, "Pump Direction (0:Infuse)"=w707, "Flow Rate (5.00)"=w703, "Flow Rate Units (1:ml/min)"=w706) -> ("VISA resource name out"=w708:refnum<visa-resource-name>)  [unwired: 10 in, 1 out]
                                n497 = call <instrlib>:"Start Pump.vi"("Run Direction (0:Infuse)"=w705, "VISA resource name"=w708) -> ()  [unwired: 8 in, 2 out]
                                }
                                }
                                }
                                }
                                n498 = case shown="False" w682 {
                                tunnel: w690 -> [w712 w714]
                                tunnel: w685 -> [_ w715]
                                frame False {
                                n499 = call "PumpStop.vi"("Pump Address"="g", "Pump COMM Port"=w712) -> ()  [unwired: 9 in, 1 out]
                                }
                                frame True {
                                n500 = call "PumpDispense.vi"("Flowrate(ul/min)"=w715, "Pump Address"="g", "Pump COMM Port"=w714) -> ()  [unwired: 7 in, 2 out]
                                }
                                }
                                n501 = case shown="True" w665 {
                                tunnel: w667 -> [_ w711]
                                frame False {
                                n502 = local write "Temperature Control 1"(FALSE) -> ()
                                }
                                frame True {
                                n503 = local write "Temperature SP 1"(w711) -> ()
                                n504 = local write "Temperature Control 1"(TRUE ("Temperature Control 1")) -> ()
                                }
                                }
                              }
                              frame #1 {
                                # "Bay 2"
                                n505 = local read "BAY 2"() -> (w725:u16)
                                n506 = Index Array(array=w734, index=2) -> (element=w732:dbl)
                                n507 = Index Array(array=w734, index=7) -> (element=w719:dbl)
                                n508 = script code="MATLAB script"("T2_SP"=w719) -> ()  [unwired: 1 in, 1 out]
                                n509 = Greater Than 0?(x=w732) -> (x > 0?=w731:bool)
                                n510 = And(x=w731, y=w729) -> (x .and. y?=w730:bool)
                                n511 = Not Equal?(x=23.0, y=w719) -> (x != y?=w720:bool)
                                n512 = Greater Or Equal?(x=w725, y=u16 1) -> (x >= y?=w723:bool)
                                n513 = Less Or Equal?(x=w725, y=u16 4) -> (x <= y?=w728:bool)
                                n514 = And(x=w723, y=w728) -> (x .and. y?=w727:bool)
                                n515 = And(x=w727, y=w729) -> (x .and. y?=w718:bool)
                                n516 = And(x=w720, y=w718) -> (x .and. y?=w717:bool)
                                n517 = case shown="True" w717 {
                                tunnel: w719 -> [_ w743]
                                frame False {
                                n518 = local write "Temperature Control 2"(FALSE) -> ()
                                }
                                frame True {
                                n519 = local write "Temperature Control 2"(TRUE ("Temperature Control 2")) -> ()
                                n520 = local write "Temperature SP 2"(w743) -> ()
                                }
                                }
                                n521 = case shown="False" w730 {
                                tunnel: w732 -> [_ w739]
                                tunnel: w736 -> [w737 w740]
                                frame False {
                                n522 = call "PumpStop.vi"("Pump Address"="i", "Pump COMM Port"=w737) -> ()  [unwired: 9 in, 1 out]
                                }
                                frame True {
                                n523 = call "PumpDispense.vi"("Flowrate(ul/min)"=w739, "Pump Address"="i", "Pump COMM Port"=w740) -> ()  [unwired: 7 in, 2 out]
                                }
                                }
                                n524 = Wait (ms)(milliseconds to wait=u32 300) -> ()  [unwired: 1 out]
                              }
                              frame #2 {
                                # "Bay 3"
                                n525 = local read "BAY 3"() -> (w752:u16)
                                n526 = Index Array(array=w762, index=3) -> (element=w760:dbl)
                                n527 = Not Equal To 0?(x=w760) -> (x != 0?=w759:bool)
                                n528 = Index Array(array=w762, index=8) -> (element=w745:dbl)
                                n529 = script code="MATLAB script"("T3_SP"=w745) -> ()  [unwired: 1 in, 1 out]
                                n530 = Less Or Equal?(x=w752, y=u16 4) -> (x <= y?=w756:bool)
                                n531 = Greater Or Equal?(x=w752, y=u16 1) -> (x >= y?=w753:bool)
                                n532 = And(x=w753, y=w756) -> (x .and. y?=w751:bool)
                                n533 = And(x=w751, y=w757) -> (x .and. y?=w747:bool)
                                n534 = And(x=w759, y=w757) -> (x .and. y?=w758:bool)
                                n535 = Not Equal?(x=23.0, y=w745) -> (x != y?=w748:bool)
                                n536 = And(x=w748, y=w747) -> (x .and. y?=w746:bool)
                                n537 = case shown="True" w758 {
                                tunnel: w760 -> [_ w767]
                                tunnel: w764 -> [w765 w768]
                                frame False {
                                n538 = call "PumpStop.vi"("Pump Address"="e", "Pump COMM Port"=w765) -> ()  [unwired: 9 in, 1 out]
                                }
                                frame True {
                                n539 = call "PumpDispense.vi"("Flowrate(ul/min)"=w767, "Pump Address"="e", "Pump COMM Port"=w768) -> ()  [unwired: 7 in, 2 out]
                                }
                                }
                                n540 = case shown="False" w746 {
                                tunnel: w745 -> [_ w771]
                                frame False {
                                n541 = local write "Temperature Control 3"(FALSE) -> ()
                                }
                                frame True {
                                n542 = local write "Temperature Control 3"(TRUE ("Temperature Control 3")) -> ()
                                n543 = local write "Temperature SP 3"(w771) -> ()
                                }
                                }
                                n544 = Wait (ms)(milliseconds to wait=u32 300) -> ()  [unwired: 1 out]
                              }
                              frame #3 {
                                # "Bay 4"
                                n545 = Index Array(array=w790, index=9) -> (element=w773:dbl)
                                n546 = script code="MATLAB script"("T4_SP"=w773) -> ()  [unwired: 1 in, 1 out]
                                n547 = Index Array(array=w790, index=4) -> (element=w788:dbl)
                                n548 = Not Equal To 0?(x=w788) -> (x != 0?=w787:bool)
                                n549 = local read "BAY 4"() -> (w779:u16)
                                n550 = And(x=w787, y=w785) -> (x .and. y?=w786:bool)
                                n551 = Less Or Equal?(x=w779, y=u16 4) -> (x <= y?=w784:bool)
                                n552 = Greater Or Equal?(x=w779, y=u16 1) -> (x >= y?=w781:bool)
                                n553 = And(x=w781, y=w784) -> (x .and. y?=w780:bool)
                                n554 = And(x=w780, y=w785) -> (x .and. y?=w775:bool)
                                n555 = case shown="True" w786 {
                                tunnel: w792 -> [w793 w796]
                                tunnel: w788 -> [_ w795]
                                frame False {
                                n556 = call "PumpStop.vi"("Pump Address"="j", "Pump COMM Port"=w793) -> ()  [unwired: 9 in, 1 out]
                                }
                                frame True {
                                n557 = call "PumpDispense.vi"("Flowrate(ul/min)"=w795, "Pump Address"="j", "Pump COMM Port"=w796) -> ()  [unwired: 7 in, 2 out]
                                }
                                }
                                n558 = Not Equal?(x=23.0, y=w773) -> (x != y?=w776:bool)
                                n559 = And(x=w776, y=w775) -> (x .and. y?=w774:bool)
                                n560 = case shown="True" w774 {
                                tunnel: w773 -> [_ w799]
                                frame False {
                                n561 = local write "Temperature Control 4"(FALSE ("Temperature Control 4")) -> ()
                                }
                                frame True {
                                n562 = local write "Temperature SP 4"(w799) -> ()
                                n563 = local write "Temperature Control 4"(TRUE ("Temperature Control 5")) -> ()
                                }
                                }
                                n564 = Wait (ms)(milliseconds to wait=u32 300) -> ()  [unwired: 1 out]
                              }
                              frame #4 {
                                # "Bay 5"
                                n565 = Index Array(array=w817, index=5) -> (element=w816:dbl)
                                n566 = Index Array(array=w817, index=4) -> (element=w804:dbl)
                                n567 = script code="MATLAB script"("T5_SP"=w804) -> ()  [unwired: 1 in, 1 out]
                                n568 = local read "BAY 5"() -> (w808:u16)
                                n569 = Not Equal To 0?(x=w816) -> (x != 0?=w815:bool)
                                n570 = And(x=w815, y=w813) -> (x .and. y?=w814:bool)
                                n571 = Less Or Equal?(x=w808, y=u16 4) -> (x <= y?=w812:bool)
                                n572 = Greater Or Equal?(x=w808, y=u16 1) -> (x >= y?=w809:bool)
                                n573 = case shown="False" w814 {
                                tunnel: w820 -> [w821 w824]
                                tunnel: w816 -> [_ w823]
                                frame False {
                                n574 = call "PumpStop.vi"("Pump Address"="h", "Pump COMM Port"=w821) -> ()  [unwired: 9 in, 1 out]
                                }
                                frame True {
                                n575 = call "PumpDispense.vi"("Flowrate(ul/min)"=w823, "Pump Address"="h", "Pump COMM Port"=w824) -> ()  [unwired: 7 in, 2 out]
                                }
                                }
                                n576 = And(x=w809, y=w812) -> (x .and. y?=w807:bool)
                                n577 = And(x=w807, y=w813) -> (x .and. y?=w802:bool)
                                n578 = Not Equal?(x=23.0, y=w804) -> (x != y?=w803:bool)
                                n579 = And(x=w803, y=w802) -> (x .and. y?=w801:bool)
                                n580 = case shown="True" w801 {
                                tunnel: w804 -> [_ w827]
                                frame False {
                                n581 = local write "Temperature Control 5"(FALSE ("Temperature Control 5")) -> ()
                                }
                                frame True {
                                n582 = local write "Temperature SP 5"(w827) -> ()
                                n583 = local write "Temperature Control 5"(TRUE ("Temperature Control 5")) -> ()
                                }
                                }
                                n584 = Wait (ms)(milliseconds to wait=u32 300) -> ()  [unwired: 1 out]
                              }
                            }
                          }
                          frame #1 {
                            # "Wait till Steady State temperature readings on all bays"
                            n585 = while {
                              tunnel: w830 -> [w831]
                              stop <- w832 stop-if-true
                              n586 = flat-sequence {
                                tunnel: [w835] -> w832
                                tunnel: w831 -> [w834]
                                frame #0 {
                                n587 = Wait (ms)(milliseconds to wait=u32 1500) -> ()  [unwired: 1 out]
                                }
                                frame #1 {
                                n588 = local read "Temp SS? 2"() -> (w838:bool)
                                n589 = local read "Temp SS? 3"() -> (w839:bool)
                                n590 = local read "Temp SS? 4"() -> (w840:bool)
                                n591 = local read "Temp SS? 5"() -> (w841:bool)
                                n592 = local read "Temp SS? 1"() -> (w837:bool)
                                n593 = Not(x=w834) -> (.not. x?=w847:bool)
                                n594 = local read "Stop"() -> (w836:bool)
                                n595 = And(x=w839, y=w840) -> (x .and. y?=w843:bool)
                                n596 = And(x=w837, y=w838) -> (x .and. y?=w844:bool)
                                n597 = And(x=w844, y=w843) -> (x .and. y?=w842:bool)
                                n598 = And(x=w842, y=w841) -> (x .and. y?=w845:bool)
                                n599 = Or(x=w847, y=w845) -> (x .or. y?=w846:bool)
                                n600 = Or(x=w846, y=w836) -> (x .or. y?=w835:bool)
                                }
                              }
                            }
                            n601 = local write "Calculate condition"(TRUE ("Calculate condition")) -> ()
                          }
                          frame #2 {
                            n602 = flat-sequence {
                              tunnel: w850 -> [w852]
                              tunnel: [w852] -> w849
                              tunnel: w849 -> [w859]
                              tunnel: [w859] -> w848
                              frame #0 {
                                n603 = local write "Equlibrating Temperature"(TRUE) -> ()
                              }
                              frame #1 {
                                # "Wait 1.5 system volumes"
                                n604 = local read "Number of System Flushes per condtion"() -> (w856:dbl)
                                n605 = local read "Extra system dead volume"() -> (w857:dbl)
                                n606 = script code="start = tic;\nP_tot = P1+P2+P3+P4+P5+P6;\nif P_tot >0\n  extra_res = extr_sys_dead_vol/P_tot;\nelse\n   extra_res =0;\nend\ntotal_sys_res = tau1 + tau2 + tau3 + tau4 + tau5 + extra_res;\ntotal_wait_time = total_sys_res*num_flush_per_cond*60;"("extr_sys_dead_vol"=w857, "num_flush_per_cond"=w856) -> ("??"=w860:errorcluster, "total_wait_time"=w854:dbl, "total_sys_res"=→"Total System Resisdence Time(min)":dbl)  [unwired: 1 in]
                                n607 = Divide(x=w854, y=60.0) -> (x/y=→"total_flush_time":dbl)
                                n608 = while {
                                tunnel: w859 -> [w862]
                                tunnel: w860 -> [w865]
                                stop <- w866 stop-if-true
                                # "Check if system is flushed every 10 seconds"
                                n609 = script code="end1 = toc(start);\nflush_time = 0;\nif end1 > total_wait_time\n   flush_time = 1;\nend\ncurr_wait_time = end1 /60;"("??"=w865) -> ("flush_time"=w869:dbl, "curr_wait_time"=w864:dbl)  [unwired: 1 out]
                                "curr_wait_time" <- w864
                                n610 = Not Equal To 0?(x=w869) -> (x != 0?=w868:bool)
                                n611 = Multiply(x=60.0, y=w864) -> ()  [unwired: 1 out]
                                n612 = local read "Stop"() -> (w871:bool)
                                n613 = Or(x=w868, y=w871) -> (x .or. y?=w867:bool)
                                n614 = Not(x=w862) -> (.not. x?=w861:bool)
                                n615 = Wait (ms)(milliseconds to wait=u32 10000) -> ()  [unwired: 1 out]
                                n616 = Or(x=w867, y=w861) -> (x .or. y?=w866:bool)
                                }
                              }
                            }
                          }
                          frame #3 {
                            # "Collect HPLC Data"
                            n617 = flat-sequence {
                              tunnel: w874 -> [w883]
                              tunnel: w873 -> [w882]
                              tunnel: w872 -> [w881]
                              tunnel: w872 -> [w880]
                              frame #0 {
                                n618 = local read "pause for ms"() -> (w877:bool)
                                n619 = case shown="True" w877 {
                                frame False {
                                }
                                frame True {
                                n620 = One Button Dialog(message="Press OK to Analyze Data", button name ("OK")="OK" ("Left Button Text (\"Yes\")")) -> ()  [unwired: 1 out]
                                }
                                }
                                n621 = local write "Flushing System"(TRUE ("Flushing System")) -> ()
                                "System Flushed?" <- TRUE ("System Flushed?")
                              }
                              frame #1 {
                                n622 = flat-sequence {
                                tunnel: w883 -> [w888]
                                tunnel: w882 -> [_]
                                tunnel: w881 -> [w887]
                                tunnel: w880 -> [w886]
                                frame #0 {
                                }
                                frame #1 {
                                n623 = flat-sequence {
                                tunnel: w888 -> [w890]
                                tunnel: w887 -> [w967]
                                tunnel: w888 -> [_]
                                tunnel: [w987] -> w885
                                tunnel: [w986] -> w884
                                tunnel: w886 -> [w985]
                                tunnel: w885 -> [w1020]
                                tunnel: w884 -> [w1019]
                                frame #0 {
                                n624 = local read "COMM Port :: Milligat Pumps"() -> (w892:refnum<visa-resource-name>)
                                n625 = stacked-sequence {
                                tunnel: w892 -> [w900 w912 w930 w935 w944 w957]
                                tunnel: w890 -> [w899 w908 w927 w937 w946 w953]
                                tunnel: 1.0 ("Flowrate(ul/min)") -> [w898 w907 w925 w934 w943 w952]
                                frame #0 {
                                n626 = Index Array(array=w899, index=0) -> (element=w902:dbl)
                                n627 = Greater Than 0?(x=w902) -> (x > 0?=w901:bool)
                                n628 = case shown="True" w901 {
                                tunnel: w900 -> [_ w905]
                                tunnel: w898 -> [_ w904]
                                frame False {
                                }
                                frame True {
                                n629 = call "PumpDispense.vi"("Flowrate(ul/min)"=w904, "Pump Address"="g", "Pump COMM Port"=w905) -> ()  [unwired: 7 in, 2 out]
                                }
                                }
                                }
                                frame #1 {
                                n630 = Index Array(array=w908, index=1) -> (element=w910:dbl)
                                n631 = Greater Than 0?(x=w910) -> (x > 0?=w909:bool)
                                n632 = case shown="True" w909 {
                                tunnel: w907 -> [_ w914]
                                tunnel: w912 -> [_ w913]
                                frame False {
                                }
                                frame True {
                                n633 = local read "Syringe_pump?"() -> (w915:bool)
                                n634 = case shown="False" w915 {
                                tunnel: w914 -> [w916 _]
                                tunnel: w913 -> [w917 _]
                                frame False {
                                n635 = call "PumpDispense.vi"("Flowrate(ul/min)"=w916, "Pump Address"="f", "Pump COMM Port"=w917) -> ()  [unwired: 7 in, 2 out]
                                }
                                frame True {
                                w924 = u16 0 items=["Infuse", "Withdraw"] ("Run Direction (0:Infuse)")
                                w920 = u32 4 items=["milliliters per hour (ml/hr)", "milliliters per minute (ml/min)", "milliliters per second (ml/sec)", "microliters per hour (ul/hr)", "microliters per minute (ul/min)", "microliters per second (ul/sec)", "nanoliters per hour (nl/hr)", "nanoliters per minute (nl/min)", "nanoliters per second (nl/sec)", "picoliters per hour (pl/hr)", "picoliters per minute (pl/min)", "picoliters per second (pl/sec)"] ("Flow Rate Units (1:ml/min)")
                                w921 = u16 0 items=["Infuse", "Withdraw"] ("Pump Direction (0:Infuse)")
                                n636 = local read "COMM Port:: Harvard Syringe Pump"() -> (w922:refnum<visa-resource-name>)
                                n637 = call <instrlib>:"Configure Flow Rate & Direction.vi"("VISA resource name"=w922, "Pump Direction (0:Infuse)"=w921, "Flow Rate (5.00)"=i8 2 ("Pump Address"), "Flow Rate Units (1:ml/min)"=w920) -> ("VISA resource name out"=w923:refnum<visa-resource-name>)  [unwired: 10 in, 1 out]
                                n638 = call <instrlib>:"Start Pump.vi"("Run Direction (0:Infuse)"=w924, "VISA resource name"=w923) -> ()  [unwired: 8 in, 2 out]
                                }
                                }
                                }
                                }
                                }
                                frame #2 {
                                n639 = Index Array(array=w927, index=2) -> (element=w928:dbl)
                                n640 = Greater Than 0?(x=w928) -> (x > 0?=w926:bool)
                                n641 = case shown="True" w926 {
                                tunnel: w930 -> [_ w932]
                                tunnel: w925 -> [_ w931]
                                frame False {
                                }
                                frame True {
                                n642 = call "PumpDispense.vi"("Flowrate(ul/min)"=w931, "Pump Address"="i", "Pump COMM Port"=w932) -> ()  [unwired: 7 in, 2 out]
                                }
                                }
                                }
                                frame #3 {
                                n643 = Index Array(array=w937, index=3) -> (element=w938:dbl)
                                n644 = Greater Than 0?(x=w938) -> (x > 0?=w936:bool)
                                n645 = case shown="True" w936 {
                                tunnel: w935 -> [_ w941]
                                tunnel: w934 -> [_ w940]
                                frame False {
                                }
                                frame True {
                                n646 = call "PumpDispense.vi"("Flowrate(ul/min)"=w940, "Pump Address"="e", "Pump COMM Port"=w941) -> ()  [unwired: 7 in, 2 out]
                                }
                                }
                                }
                                frame #4 {
                                n647 = Index Array(array=w946, index=4) -> (element=w947:dbl)
                                n648 = Greater Than 0?(x=w947) -> (x > 0?=w945:bool)
                                n649 = case shown="True" w945 {
                                tunnel: w944 -> [_ w950]
                                tunnel: w943 -> [_ w949]
                                frame False {
                                }
                                frame True {
                                n650 = call "PumpDispense.vi"("Flowrate(ul/min)"=w949, "Pump Address"="j", "Pump COMM Port"=w950) -> ()  [unwired: 7 in, 2 out]
                                }
                                }
                                }
                                frame #5 {
                                n651 = Index Array(array=w953, index=5) -> (element=w955:dbl)
                                n652 = Greater Than 0?(x=w955) -> (x > 0?=w954:bool)
                                n653 = case shown="True" w954 {
                                tunnel: w957 -> [_ w959]
                                tunnel: w952 -> [_ w958]
                                frame False {
                                }
                                frame True {
                                n654 = call "PumpDispense.vi"("Flowrate(ul/min)"=w958, "Pump Address"="h", "Pump COMM Port"=w959) -> ()  [unwired: 7 in, 2 out]
                                }
                                }
                                }
                                }
                                n655 = stacked-sequence {
                                tunnel: FALSE -> [w893 w894 w895 w896 w897]
                                frame #0 {
                                n656 = local write "Temperature Control 1"(w893) -> ()
                                }
                                frame #1 {
                                n657 = local write "Temperature Control 2"(w894) -> ()
                                }
                                frame #2 {
                                n658 = local write "Temperature Control 3"(w895) -> ()
                                }
                                frame #3 {
                                n659 = local write "Temperature Control 4"(w896) -> ()
                                }
                                frame #4 {
                                n660 = local write "Temperature Control 5"(w897) -> ()
                                }
                                }
                                }
                                frame #1 {
                                n661 = while {
                                stop <- w966 stop-if-true
                                n662 = local read "Phase_Sensor_voltage"() -> (w961:dbl)
                                n663 = script code="organic_phase = 0;\nif start_phase_time \n   start_phase_timer = tic;\n   start_phase_time = 0;\nelse\n  %ignore phase sensor values\n  %if not(phase_sensor_val >2.9 && phase_sensor_val <3.8)\n    %    start_phase_timer = tic;\n   %end\n\n   end_phase_time =  toc(start_phase_timer )\n\n   if end_phase_time > 2\n       organic_phase = 1;\n       start_phase_time = 1;\n   end\n\nend"("phase_sensor_val"=w961) -> ("organic_phase"=w963:dbl)  [unwired: 1 in, 1 out]
                                n664 = local read "Stop"() -> (w965:bool)
                                n665 = Not Equal To 0?(x=w963) -> (x != 0?=w964:bool)
                                n666 = Or(x=w964, y=w965) -> (x .or. y?=w966:bool)
                                n667 = Wait (ms)(milliseconds to wait=u32 300) -> ()  [unwired: 1 out]
                                }
                                }
                                frame #2 {
                                n668 = local read "Stop"() -> (w969:bool)
                                n669 = Not(x=w969) -> (.not. x?=w968:bool)
                                n670 = local read "Sample Valve COMM::Port"() -> (w970:refnum<visa-resource-name>)
                                n671 = case shown="True" w968 {
                                tunnel: w970 -> [_ w972]
                                tunnel: w967 -> [_ w971]
                                frame False {
                                }
                                frame True {
                                n672 = flat-sequence {
                                tunnel: w971 -> [w974]
                                tunnel: w972 -> [w984]
                                frame #0 {
                                n673 = local read "Sample Valve COMM::Port"() -> (w973:refnum<visa-resource-name>)
                                n674 = flat-sequence {
                                tunnel: w976 -> [w981]
                                tunnel: [w981] -> w975
                                frame #0 {
                                n675 = Wait (ms)(milliseconds to wait=u32 500) -> ()  [unwired: 1 out]
                                }
                                }
                                n676 = call-poly <vilib>:"Digital Write.vi"("Output Value"=FALSE, "DO Channel"=u8 22, "LINX Resource"=w975) -> ()  [unwired: 7 in, 2 out]
                                n677 = call-poly <vilib>:"Digital Write.vi"("Output Value"=TRUE, "DO Channel"=u8 22, "LINX Resource"=w974) -> ("LINX Resource"=w976:T10)  [unwired: 7 in, 1 out]
                                n678 = call "NanoValve Inject.vi"("VISA resource name"=w973) -> ()  [unwired: 10 in, 1 out]
                                }
                                frame #1 {
                                n679 = Wait (ms)(milliseconds to wait=u32 2000) -> ()  [unwired: 1 out]
                                }
                                frame #2 {
                                n680 = call "NanoValve Load.vi"("VISA resource name"=w984) -> ()  [unwired: 10 in, 1 out]
                                }
                                }
                                }
                                }
                                }
                                frame #3 {
                                n681 = local read "Stop"() -> (w990:bool)
                                n682 = local read "Bay Parameters"() -> (w986:T2)
                                n683 = Unbundle By Name(w986) -> ("Hplc Wait time(min)"=w988:dbl)
                                n684 = Not(x=w990) -> (.not. x?=w989:bool)
                                n685 = case shown="True" w989 {
                                tunnel: w988 -> [_ w995]
                                tunnel: [errorcluster {"status"=FALSE, "code"=0, "source"=""} ("error out") w994] -> w987
                                tunnel: w986 -> [_ w993]
                                tunnel: w985 -> [_ w992]
                                frame False {
                                }
                                frame True {
                                n686 = flat-sequence {
                                tunnel: w995 -> [w997]
                                tunnel: w992 -> [w1006]
                                tunnel: [w1017] -> w994
                                tunnel: w993 -> [w1016]
                                frame #0 {
                                # "Wait till for HPLC Method"
                                n687 = script code="start = tic;"() -> ("??"=w996:errorcluster)  [unwired: 1 in]
                                n688 = while {
                                tunnel: w997 -> [w999]
                                tunnel: w996 -> [w998]
                                stop <- w1005 stop-if-true
                                n689 = Multiply(x=w999, y=60.0) -> (x*y=w1000:dbl)
                                n690 = script code="end1 = toc(start);\nflush_time = 0;\nif end1 > hplc_wait_time\n   flush_time = 1;\nend"("??"=w998, "hplc_wait_time"=w1000) -> ("flush_time"=w1002:dbl)  [unwired: 1 out]
                                n691 = local read "Stop"() -> (w1004:bool)
                                n692 = Not Equal To 0?(x=w1002) -> (x != 0?=w1003:bool)
                                n693 = Or(x=w1003, y=w1004) -> (x .or. y?=w1005:bool)
                                }
                                }
                                frame #1 {
                                n694 = flat-sequence {
                                tunnel: w1008 -> [w1013]
                                tunnel: [w1013] -> w1007
                                frame #0 {
                                n695 = Wait (ms)(milliseconds to wait=u32 500) -> ()  [unwired: 1 out]
                                }
                                }
                                n696 = call-poly <vilib>:"Digital Write.vi"("Output Value"=FALSE, "DO Channel"=u8 24, "LINX Resource"=w1006) -> ("LINX Resource"=w1008:T10)  [unwired: 7 in, 1 out]
                                n697 = call-poly <vilib>:"Digital Write.vi"("Output Value"=TRUE, "DO Channel"=u8 24, "LINX Resource"=w1007) -> ()  [unwired: 7 in, 2 out]
                                }
                                frame #2 {
                                n698 = Wait (ms)(milliseconds to wait=u32 30000) -> ()  [unwired: 1 out]
                                }
                                frame #3 {
                                n699 = Unbundle By Name(w1016) -> ("hplc File Name"=w1018:string)
                                n700 = call "hplc_analyze.vi"("File Path"=w1018) -> ("error out"=w1017:errorcluster)  [unwired: 10 in]
                                }
                                }
                                }
                                }
                                }
                                frame #4 {
                                n701 = Unbundle By Name(w1020) -> ("status"=w1021:bool)
                                n702 = case shown="False" w1021 {
                                tunnel: w1019 -> [_ w1022]
                                frame False {
                                }
                                frame True {
                                n703 = while {
                                tunnel: w1022 -> [w1024]
                                stop <- w1023 stop-if-true
                                w1029 = "An error occured while trying to read HPLC data. " ("message")
                                n704 = local write "Error Message"(w1029) -> ()
                                n705 = call <vilib>:"Three Button Dialog.vi"("Right Button Text (\"Cancel\")"="STOP EXPs" ("F button name (\"Cancel\")"), "Center Button Text (\"No\")"="REDO" ("T button name (\"OK\")"), "Left Button Text (\"Yes\")"="REREAD" ("T button name (\"OK\")"), "message"=w1029) -> ("Which Button?"=w1025:T19)  [unwired: 7 in]
                                n706 = case shown="\"Left Button\"" w1025 {
                                tunnel: w1024 -> [_ _ w1036 _]
                                tunnel: [TRUE TRUE w1035 w1038] -> w1023
                                frame "Right Button" {
                                w1030 = TRUE ("Setup Error")
                                n707 = local write "System Error"(w1030) -> ()
                                n708 = local write "Setup Error"(w1030) -> ()
                                n709 = script code="system_error = 1"() -> ()  [unwired: 1 in, 1 out]
                                n710 = local write "Stop"(w1030) -> ()
                                }
                                frame "Center Button" {
                                n711 = script code="redo = true;\nopt_ctr = 1;\nCurrExp = CurrExp + 1;\nncall0 = ncall0 +1;\nif req_ctr == req_tot\n       opt_ctr = 3;\n  else\n     req_ctr = req_ctr +1;\nend"() -> ()  [unwired: 1 in, 1 out]
                                }
                                frame "Left Button" {
                                n712 = Unbundle By Name(w1036) -> ("hplc File Name"=w1037:string)
                                n713 = call "hplc_analyze.vi"("File Path"=w1037) -> ("error out"=w1033:errorcluster)  [unwired: 10 in]
                                n714 = Unbundle By Name(w1033) -> ("status"=w1034:bool)
                                n715 = Not(x=w1034) -> (.not. x?=w1035:bool)
                                }
                                frame "Window Close" {
                                w1038 = TRUE
                                n716 = local write "Setup Error"(w1038) -> ()
                                n717 = script code="system_error = 1"() -> ()  [unwired: 1 in, 1 out]
                                n718 = local write "Stop"(w1038) -> ()
                                }
                                }
                                }
                                }
                                }
                                }
                                frame #5 {
                                n719 = disable-structure shown="Disabled" {
                                frame Disabled {
                                n720 = flat-sequence {
                                tunnel: w1040 -> [w1045]
                                tunnel: [w1045] -> w1039
                                frame #0 {
                                n721 = Wait (ms)(milliseconds to wait=u32 500) -> ()  [unwired: 1 out]
                                }
                                }
                                n722 = call-poly <vilib>:"Digital Write.vi"("Output Value"=FALSE, "DO Channel"=u8 22) -> ("LINX Resource"=w1040:T10)  [unwired: 8 in, 1 out]
                                n723 = call-poly <vilib>:"Digital Write.vi"("Output Value"=TRUE, "DO Channel"=u8 22, "LINX Resource"=w1039) -> ()  [unwired: 7 in, 2 out]
                                }
                                frame Enabled {
                                }
                                }
                                }
                                }
                                }
                                }
                              }
                              frame #2 {
                                n724 = local read "Stop"() -> (w1048:bool)
                                n725 = local write "HPLC Analysis"(TRUE ("HPLC Analysis")) -> ()
                                n726 = Not(x=w1048) -> (.not. x?=w1047:bool)
                                n727 = case shown="True" w1047 {
                                frame False {
                                }
                                frame True {
                                n728 = script code="C_measured =Conc;\nFvalues(end +1,:) = [Conc];"() -> ()  [unwired: 1 in, 1 out]
                                }
                                }
                              }
                            }
                          }
                          frame #4 {
                            n729 = local read "Stop"() -> (w1051:bool)
                            n730 = Not(x=w1051) -> (.not. x?=w1050:bool)
                            n731 = case shown="True" w1050 {
                              tunnel: [1.0 w1062] -> w1052
                              frame False {
                              }
                              frame True {
                                # "Save data to excel file"
                                n732 = local read "Bay Parameters"() -> (w1060:T2)
                                n733 = Unbundle By Name(w1060) -> ("Total Number of Experiments 2"=w1059:dbl)
                                n734 = script code="analyze_labview_results"("ncall"=w1059) -> ("terminate"=w1062:dbl, "ncall0"=w1061:dbl, "experiment_history"=w1057:dbl[][], "Pbest"=w1055:dbl[], "Tbest"=w1056:dbl[], "best_exp_num"=w1054:dbl)  [unwired: 1 in, 1 out]
                                n735 = local write "Flowrates(ul/min)_best"(w1055) -> ()
                                n736 = local write "temperature_best"(w1056) -> ()
                                n737 = local write "best_exp_num"(w1054) -> ()
                                n738 = local write "Current Experiment"(w1061) -> ()
                                n739 = local write "Total Number of Experiments"(w1059) -> ()
                                n740 = call-poly <vilib>:"Array To Matrix.vi"("Real 2D Array"=w1057) -> ("Real Matrix"=w1058:T18)
                                n741 = local write "experiment history"(w1058) -> ()
                              }
                            }
                          }
                          frame #5 {
                            n742 = local read "Num_exp_till_pause"() -> (w1064:i32)
                            n743 = Increment(x=w1064) -> (x+1=w1063:i32)
                            n744 = local write "Num_exp_till_pause"(w1063) -> ()
                          }
                          frame #6 {
                            # "Pause System"
                            n745 = local read "Bay Parameters"() -> (w1072:T2)
                            n746 = Unbundle By Name(w1072) -> ("Num_conditons_per_wait"=w1071:dbl)
                            n747 = local read "Num_exp_till_pause"() -> (w1070:i32)
                            n748 = Equal?(x=w1071, y=w1070) -> (x = y?=w1069:bool)
                            n749 = local read "Run_Stop_cluster"() -> (w1066:T7)
                            n750 = Unbundle By Name(w1066) -> ("Stop Run Button"=w1068:bool)
                            n751 = Or(x=w1068, y=w1069) -> (x .or. y?=w1067:bool)
                            n752 = case shown="True" w1067 {
                              tunnel: w1071 -> [w1075 _]
                              tunnel: w1070 -> [w1076 _]
                              tunnel: w1066 -> [_ w1078]
                              frame False {
                                n753 = Greater?(x=w1076, y=w1075) -> (0:w1074:bool)
                                n754 = case shown="True" w1074 {
                                frame False {
                                }
                                frame True {
                                n755 = local write "Num_exp_till_pause"(0 ("Num_exp_till_pause")) -> ()
                                }
                                }
                              }
                              frame True {
                                n756 = flat-sequence {
                                tunnel: w1078 -> [w1106]
                                frame #0 {
                                w1082 = string[] ["e", "f", "g", "h", "i", "j"]
                                # "Turn off pumps and stop controling temperature"
                                n757 = stacked-sequence {
                                frame #0 {
                                n758 = local write "Temperature Control 1"(FALSE ("Temperature Control 1")) -> ()
                                }
                                frame #1 {
                                n759 = local write "Temperature Control 2"(FALSE ("Temperature Control 2")) -> ()
                                }
                                frame #2 {
                                n760 = local write "Temperature Control 3"(FALSE ("Temperature Control 3")) -> ()
                                }
                                frame #3 {
                                n761 = local write "Temperature Control 4"(FALSE ("Temperature Control 4")) -> ()
                                }
                                frame #4 {
                                n762 = local write "Temperature Control 5"(FALSE ("Temperature Control 5")) -> ()
                                }
                                }
                                n763 = local read "COMM Port:: Harvard Syringe Pump"() -> (w1080:refnum<visa-resource-name>)
                                n764 = local read "Syringe_pump?"() -> (w1079:bool)
                                n765 = local read "COMM Port :: Milligat Pumps"() -> (w1081:refnum<visa-resource-name>)
                                n766 = Array Size(array=w1082) -> (size(s)=w1083:i32)
                                n767 = case shown="True" w1079 {
                                tunnel: w1080 -> [_ w1091]
                                frame False {
                                }
                                frame True {
                                n768 = call <instrlib>:"Stop Pump.vi"("VISA resource name"=w1091) -> ()  [unwired: 9 in, 2 out]
                                }
                                }
                                n769 = for {
                                N: w1083 -> [_]
                                tunnel: w1082 -> [w1089] mode=indexing
                                tunnel: w1081 -> [w1090]
                                n770 = call "PumpStop.vi"("Pump Address"=w1089, "Pump COMM Port"=w1090) -> ()  [unwired: 9 in, 1 out]
                                }
                                }
                                frame #1 {
                                n771 = local read "Stop"() -> (w1094:bool)
                                n772 = Not(x=w1094) -> (.not. x?=w1093:bool)
                                n773 = case shown="True" w1093 {
                                frame False {
                                }
                                frame True {
                                n774 = while {
                                stop <- w1100 stop-if-true
                                # "Wait till user confirms system resume"
                                n775 = Two Button Dialog(message="System is currently paused. Refill Syringes, flush lines, then press OK to continue optimization.\nOr Redo to repeat condition ", 1:"REDO" ("F button name (\"Cancel\")"), 2:"OK" ("Left Button Text (\"Yes\")")) -> (T button?=w1096:bool)
                                n776 = case shown="False" w1096 {
                                tunnel: [TRUE TRUE] -> w1095
                                frame False {
                                n777 = script code="redo = true;"() -> ()  [unwired: 1 in, 1 out]
                                }
                                frame True {
                                }
                                }
                                n778 = local read "Stop"() -> (w1101:bool)
                                n779 = Or(x=w1095, y=w1101) -> (x .or. y?=w1100:bool)
                                }
                                }
                                }
                                n780 = local write "stop_xl_write"(TRUE ("stop_xl_write")) -> ()
                                }
                                frame #2 {
                                n781 = local write "Num_exp_till_pause"(0 ("Num_exp_till_pause")) -> ()
                                n782 = Bundle By Name(cluster=w1106, "Stop Run Button"=FALSE) -> (w1104:T7)
                                n783 = local write "Run_Stop_cluster"(w1104) -> ()
                                }
                                }
                              }
                            }
                          }
                          frame #7 {
                            w1109 = FALSE
                            n784 = local write "Equlibrating Temperature"(w1109) -> ()
                            n785 = local write "Calculate condition"(w1109) -> ()
                            n786 = local write "Flushing System"(w1109) -> ()
                            n787 = local write "HPLC Analysis"(w1109) -> ()
                            n788 = local write "stop_xl_write"(TRUE ("stop_xl_write")) -> ()
                          }
                        }
                        n789 = while {
                          stop <- w1136 stop-if-true
                          n790 = flat-sequence {
                            frame #0 {
                              n791 = script code="save_excel_time_data;"() -> ()  [unwired: 1 in, 1 out]
                            }
                            frame #1 {
                              n792 = Wait (ms)(milliseconds to wait=u32 30000) -> ()  [unwired: 1 out]
                            }
                          }
                          n793 = local read "Stop"() -> (w1137:bool)
                          n794 = local read "stop_xl_write"() -> (w1135:bool)
                          n795 = Or(x=w1135, y=w1137) -> (x .or. y?=w1136:bool)
                        }
                      }
                    }
                  }
                }
                n796 = Greater?(x=w602, y=w603) -> (0:w610:bool)
                n797 = Equal?(x=w608, y=1.0) -> (x = y?=w604:bool)
                n798 = local read "Stop"() -> (w611:bool)
                n799 = Or(x=w611, y=w610) -> (x .or. y?=w607:bool)
                n800 = Or(x=w604, y=w607) -> (x .or. y?=w606:bool)
                n801 = case shown="True" w604 {
                  frame False {
                  }
                  frame True {
                    w615 = u16 2 items=["System  Error", "System Running", "System Standby"] ("System Status")
                    n802 = local write "Stop"(TRUE ("Stop")) -> ()
                    n803 = local write "System Status"(w615) -> ()
                  }
                }
                "Optimization_loop_index" <- w612
              }
            }
          }
          n804 = while {
            tunnel: w590 -> [w1232]
            stop <- w1235 stop-if-true
            n805 = local read "Temperature Control 3"() -> (w1233:bool)
            n806 = local read "running?"() -> (w1231:bool)
            n807 = And(x=w1231, y=w1233) -> (x .and. y?=w1234:bool)
            n808 = case shown="True" w1234 {
              tunnel: w1232 -> [_ w1238]
              frame False {
                n809 = local write "Temp SS? 3"(TRUE) -> ()
              }
              frame True {
                # "Bay 3 Temperature Controller"
                n810 = local read "Temperature SP 3"() -> (w1239:dbl)
                n811 = local read "Temperature 3"() -> (w1242:dbl)
                n812 = Subtract(x=w1242, y=w1239) -> (x-y=w1251:dbl)
                n813 = Absolute Value(x=w1251) -> (abs(x)=w1253:dbl)
                n814 = Less Or Equal?(x=w1253, y=1.2) -> (x <= y?=w1250:bool)
                n815 = local write "Temp SS? 3"(w1250) -> ()
                n816 = local read "SSR Duration 3"() -> (w1260:dbl)
                n817 = call-poly <vilib>:"PID Online Autotuning.vi"("setpoint"=w1239, "manipulated variable"=w1260, "autotuning parameters"=T9 {"type of controller"=enum."PID", "relay cycles"=3, "relay amplitude"=1.0, "control specifications"=enum."Normal", "PV noise level"=0.1} ("Autotuning Parameters R1"), "process variable"=w1242, "PID gains in"=T8 {"Proportional gain Kc"=0.38538, "Integral time Ti (sec)"=0.524375, "Derivative time Ti (sec)"=0.12585} ("PID gains 2")) -> ("setpoint out"=w1258:dbl, "process variable out"=w1259:dbl, "PID gains out"=w1262:T17)  [unwired: 6 in, 2 out]
                n818 = Greater?(x=w1239, y=w1242) -> (0:w1249:bool)
                n819 = call <vilib>:"PID Autotuning (Temperature).vi"("desired temperature"=w1258, "measured temperature"=w1259, "PID gains in"=w1262, "output range"=cluster{"output high":dbl, "output low":dbl} {"output high"=3.0, "output low"=-1.0} ("Output range")) -> ("output"=w1255:dbl)  [unwired: 12 in, 3 out]
                n820 = Multiply(x=1000.0, y=w1255) -> (x*y=w1257:dbl)
                n821 = local write "SSR Duration 3"(w1255) -> ()
                n822 = Greater Than 0?(x=w1257) -> (x > 0?=w1248:bool)
                n823 = And(x=w1248, y=w1249) -> (x .and. y?=w1246:bool)
                n824 = Subtract(x=w1242, y=10.0) -> (x-y=w1244:dbl)
                n825 = Less?(x=w1244, y=w1239) -> (x < y?=w1247:bool)
                n826 = And(x=w1247, y=w1246) -> (x .and. y?=w1245:bool)
                n827 = case shown="True" w1245 {
                  tunnel: [errorcluster {"status"=FALSE, "code"=0, "source"=""} ("error out") w1274] -> _
                  tunnel: 4 -> [_ w1272]
                  tunnel: w1257 -> [w1268 w1273]
                  tunnel: [0.0 w1276] -> w1240
                  tunnel: w1239 -> [_ w1275]
                  tunnel: w1238 -> [_ w1271]
                  frame False {
                    n828 = Absolute Value(x=w1268) -> (abs(x)=w1269:dbl)
                    n829 = Wait (ms)(milliseconds to wait=w1269) -> ()  [unwired: 1 out]
                  }
                  frame True {
                    n830 = call "TurnOnRelayArduino.vi"("channel"=w1272, "duration"=w1273, "LINX Resource"=w1271) -> ("error out"=w1274:errorcluster)  [unwired: 7 in, 1 out]
                    n831 = script code="tempdiff3= SP3 - T3;\nif tempdiff3 > 10\n  if slope3 < .01\n     temp_check3 = temp_check3 + 1;\n  else\n      temp_check3 =0;\n  end\nend\n\nif temp_check3 > 9\n  temp_error3 = 1\nend"("SP3"=w1275) -> ("temp_error3"=w1276:dbl)  [unwired: 1 in, 1 out]
                  }
                }
                n832 = Not Equal To 0?(x=w1240) -> (x != 0?=w1241:bool)
                n833 = case shown="True" w1241 {
                  frame False {
                  }
                  frame True {
                    n834 = local write "Error Message"("Bay 3 Temperature Heating Error") -> ()
                  }
                }
                n835 = case shown="True" w1241 {
                  tunnel: w1241 -> [_ w1266]
                  frame False {
                  }
                  frame True {
                    n836 = local write "System Error"(w1266) -> ()
                    n837 = local write "Stop"(w1266) -> ()
                  }
                }
              }
            }
            n838 = Wait (ms)(milliseconds to wait=u32 400) -> ()  [unwired: 1 out]
            n839 = local read "Stop"() -> (w1235:bool)
          }
          n840 = while {
            tunnel: w590 -> [w1186]
            stop <- w1189 stop-if-true
            n841 = local read "running?"() -> (w1185:bool)
            n842 = Wait (ms)(milliseconds to wait=u32 400) -> ()  [unwired: 1 out]
            n843 = local read "Temperature Control 4"() -> (w1188:bool)
            n844 = And(x=w1185, y=w1188) -> (x .and. y?=w1187:bool)
            n845 = case shown="True" w1187 {
              tunnel: w1186 -> [_ w1192]
              frame False {
                n846 = local write "Temp SS? 4"(TRUE ("Temp SS? 4")) -> ()
              }
              frame True {
                # "Bay 4 Temperature Controller"
                n847 = local read "Temperature SP 4"() -> (w1195:dbl)
                n848 = local read "Temperature 4"() -> (w1198:dbl)
                n849 = Subtract(x=w1198, y=w1195) -> (x-y=w1205:dbl)
                n850 = Absolute Value(x=w1205) -> (abs(x)=w1207:dbl)
                n851 = Less Or Equal?(x=w1207, y=1.2) -> (x <= y?=w1204:bool)
                n852 = local write "Temp SS? 4"(w1204) -> ()
                n853 = local read "SSR Duration 4"() -> (w1208:dbl)
                n854 = call-poly <vilib>:"PID Online Autotuning.vi"("setpoint"=w1195, "manipulated variable"=w1208, "autotuning parameters"=T9 {"type of controller"=enum."PID", "relay cycles"=3, "relay amplitude"=1.0, "control specifications"=enum."Normal", "PV noise level"=0.1} ("Autotuning Parameters R1"), "process variable"=w1198, "PID gains in"=T8 {"Proportional gain Kc"=0.38538, "Integral time Ti (sec)"=0.524375, "Derivative time Ti (sec)"=0.12585} ("PID gains 2")) -> ("setpoint out"=w1210:dbl, "process variable out"=w1211:dbl, "PID gains out"=w1213:T17)  [unwired: 6 in, 2 out]
                n855 = call <vilib>:"PID Autotuning (Temperature).vi"("desired temperature"=w1210, "measured temperature"=w1211, "PID gains in"=w1213, "output range"=cluster{"output high":dbl, "output low":dbl} {"output high"=3.0, "output low"=-1.0} ("Output range")) -> ("output"=w1209:dbl)  [unwired: 12 in, 3 out]
                n856 = Subtract(x=w1198, y=10.0) -> (x-y=w1197:dbl)
                n857 = Less?(x=w1197, y=w1195) -> (x < y?=w1199:bool)
                n858 = Multiply(x=1000.0, y=w1209) -> (x*y=w1217:dbl)
                n859 = Greater?(x=w1195, y=w1198) -> (0:w1203:bool)
                n860 = Greater Than 0?(x=w1217) -> (x > 0?=w1202:bool)
                n861 = local write "SSR Duration 4"(w1209) -> ()
                n862 = And(x=w1202, y=w1203) -> (x .and. y?=w1201:bool)
                n863 = And(x=w1199, y=w1201) -> (x .and. y?=w1200:bool)
                n864 = case shown="True" w1200 {
                  tunnel: [errorcluster {"status"=FALSE, "code"=0, "source"=""} ("error out") w1228] -> _
                  tunnel: 5 -> [_ w1226]
                  tunnel: w1217 -> [w1222 w1227]
                  tunnel: w1195 -> [_ w1230]
                  tunnel: [0.0 w1229] -> w1194
                  tunnel: w1192 -> [_ w1225]
                  frame False {
                    n865 = Absolute Value(x=w1222) -> (abs(x)=w1223:dbl)
                    n866 = Wait (ms)(milliseconds to wait=w1223) -> ()  [unwired: 1 out]
                  }
                  frame True {
                    n867 = call "TurnOnRelayArduino.vi"("channel"=w1226, "duration"=w1227, "LINX Resource"=w1225) -> ("error out"=w1228:errorcluster)  [unwired: 7 in, 1 out]
                    n868 = script code="tempdiff4= SP4 - T4;\nif tempdiff4 > 10\n  if slope4 < .01\n     temp_check4 = temp_check4 + 1;\n  else\n      temp_check4 =0;\n  end\nend\n\nif temp_check4 > 9\n  temp_error4 = 1\nend"("SP4"=w1230) -> ("temp_error4"=w1229:dbl)  [unwired: 1 in, 1 out]
                  }
                }
                n869 = Not Equal To 0?(x=w1194) -> (x != 0?=w1193:bool)
                n870 = case shown="True" w1193 {
                  frame False {
                  }
                  frame True {
                    n871 = local write "Error Message"("Bay 4 Temperature Heating Error") -> ()
                  }
                }
                n872 = case shown="True" w1193 {
                  tunnel: w1193 -> [_ w1220]
                  frame False {
                  }
                  frame True {
                    n873 = local write "System Error"(w1220) -> ()
                    n874 = local write "Stop"(w1220) -> ()
                  }
                }
              }
            }
            n875 = local read "Stop"() -> (w1189:bool)
          }
          n876 = while {
            stop <- w595 stop-if-true
            n877 = script code="TempArr1=circshift(TempArr1,9);\nTempArr2=circshift(TempArr2,9);\nTempArr3=circshift(TempArr3,9);\nTempArr4=circshift(TempArr4,9);\nTempArr5=circshift(TempArr5,9);\n\nTempArr1(10)=T1;\nTempArr2(10)=T2;\nTempArr3(10)=T3;\nTempArr4(10)=T4;\nTempArr5(10)=T5;\n\n[slope1 temp] = polyfit([1,2,3,4,5,6,7,8,9,10]',TempArr1,1);\nslope1 = slope1(1);\n[slope2 temp] = polyfit([1,2,3,4,5,6,7,8,9,10]',TempArr2,1);\nslope2= slope2(1);\n[slope3 temp] = polyfit([1,2,3,4,5,6,7,8,9,10]',TempArr3,1);\nslope3 = slope3(1);\n[slope4 temp] = polyfit([1,2,3,4,5,6,7,8,9,10]',TempArr4,1);\nslope4 = slope4(1);\n[slope5 temp] = polyfit([1,2,3,4,5,6,7,8,9,10]',TempArr5,1);\nslope5 = slope5(1);"() -> ()  [unwired: 1 in, 1 out]
            n878 = Wait (ms)(milliseconds to wait=u32 600) -> ()  [unwired: 1 out]
            n879 = local read "Stop"() -> (w595:bool)
          }
          n880 = while {
            tunnel: w590 -> [w1140]
            stop <- w1143 stop-if-true
            n881 = local read "running?"() -> (w1139:bool)
            n882 = local read "Temperature Control 5"() -> (w1141:bool)
            n883 = And(x=w1139, y=w1141) -> (x .and. y?=w1142:bool)
            n884 = case shown="True" w1142 {
              tunnel: w1140 -> [_ w1146]
              frame False {
                n885 = local write "Temp SS? 5"(TRUE ("Temp SS? 5")) -> ()
              }
              frame True {
                # "Bay 5 Temperature Controller"
                n886 = local read "SSR Duration 5"() -> (w1162:dbl)
                n887 = local read "Temperature SP 5"() -> (w1148:dbl)
                n888 = local read "Temperature 5"() -> (w1151:dbl)
                n889 = Subtract(x=w1151, y=w1148) -> (x-y=w1159:dbl)
                n890 = Absolute Value(x=w1159) -> (abs(x)=w1161:dbl)
                n891 = Less Or Equal?(x=w1161, y=1.2) -> (x <= y?=w1158:bool)
                n892 = local write "Temp SS? 5"(w1158) -> ()
                n893 = call-poly <vilib>:"PID Online Autotuning.vi"("setpoint"=w1148, "manipulated variable"=w1162, "autotuning parameters"=T9 {"type of controller"=enum."PID", "relay cycles"=3, "relay amplitude"=1.0, "control specifications"=enum."Normal", "PV noise level"=0.1} ("Autotuning Parameters R1"), "process variable"=w1151, "PID gains in"=T8 {"Proportional gain Kc"=0.38538, "Integral time Ti (sec)"=0.524375, "Derivative time Ti (sec)"=0.12585} ("PID gains 2")) -> ("setpoint out"=w1164:dbl, "process variable out"=w1165:dbl, "PID gains out"=w1167:T17)  [unwired: 6 in, 2 out]
                n894 = call <vilib>:"PID Autotuning (Temperature).vi"("desired temperature"=w1164, "measured temperature"=w1165, "PID gains in"=w1167, "output range"=cluster{"output high":dbl, "output low":dbl} {"output high"=3.0, "output low"=-1.0} ("Output range")) -> ("output"=w1163:dbl)  [unwired: 12 in, 3 out]
                n895 = Multiply(x=1000.0, y=w1163) -> (x*y=w1171:dbl)
                n896 = Greater?(x=w1148, y=w1151) -> (0:w1156:bool)
                n897 = Greater Than 0?(x=w1171) -> (x > 0?=w1157:bool)
                n898 = local write "SSR Duration 5"(w1163) -> ()
                n899 = And(x=w1157, y=w1156) -> (x .and. y?=w1154:bool)
                n900 = Subtract(x=w1151, y=10.0) -> (x-y=w1152:dbl)
                n901 = Greater?(x=w1152, y=w1148) -> (0:w1155:bool)
                n902 = And(x=w1155, y=w1154) -> (x .and. y?=w1153:bool)
                n903 = case shown="True" w1153 {
                  tunnel: [errorcluster {"status"=FALSE, "code"=0, "source"=""} ("error out") w1182] -> _
                  tunnel: 6 -> [_ w1179]
                  tunnel: w1171 -> [w1176 w1180]
                  tunnel: [0.0 w1184] -> w1149
                  tunnel: w1148 -> [_ w1183]
                  tunnel: w1146 -> [_ w1181]
                  frame False {
                    n904 = Absolute Value(x=w1176) -> (abs(x)=w1177:dbl)
                    n905 = Wait (ms)(milliseconds to wait=w1177) -> ()  [unwired: 1 out]
                  }
                  frame True {
                    n906 = call "TurnOnRelayArduino.vi"("channel"=w1179, "duration"=w1180, "LINX Resource"=w1181) -> ("error out"=w1182:errorcluster)  [unwired: 7 in, 1 out]
                    n907 = script code="tempdiff5= SP5 - T5;\n\nif tempdiff5 > 10\n  if slope5 < .01\n     temp_check5 = temp_check5 + 1;\n  else\n      temp_check5 =0;\n  end\nend\n\nif temp_check5 >9\n  temp_error5 = 1\nend"("SP5"=w1183) -> ("temp_error5"=w1184:dbl)  [unwired: 1 in, 1 out]
                  }
                }
                n908 = Not Equal To 0?(x=w1149) -> (x != 0?=w1147:bool)
                n909 = case shown="True" w1147 {
                  frame False {
                  }
                  frame True {
                    n910 = local write "Error Message"("Bay 5 Temperature Heating Error") -> ()
                  }
                }
                n911 = case shown="True" w1147 {
                  tunnel: w1147 -> [_ w1174]
                  frame False {
                  }
                  frame True {
                    n912 = local write "Stop"(w1174) -> ()
                    n913 = local write "System Error"(w1174) -> ()
                  }
                }
              }
            }
            n914 = Wait (ms)(milliseconds to wait=u32 400) -> ()  [unwired: 1 out]
            n915 = local read "Stop"() -> (w1143:bool)
          }
        }
      }
      n916 = local read "IR Sensor Device"() -> (w62:T6)
      n917 = while {
        tunnel: errorcluster {"status"=FALSE, "code"=0, "source"=""} ("error out") -> [w133]
        tunnel: w62 -> [w152]
        stop <- w173 stop-if-true
        w130 = u8 7 items=["RAM IR raw  Ch1"=4, "RAM IR raw  Ch2"=5, "RAM T_A"=6, "RAM T_OBJ1"=7, "RAM T_OBJ2"=8, "EEPROM_To_max"=32, "EEPROM_To_min"=33, "EEPROM_PWM_CTRL"=34, "EEPROM_Ta_range"=35, "EEPROM_Emissivity_CorrCoeff"=36, "EEPROM_SMBus Address"=46, "EEPROM_ConfigReg"=37] ("Melexis_Cmmds")
        # "Bay 5 Temperature Read"
        # "Bay 4 Temperature Read"
        # "Bay 3 Temperature Read"
        # "Bay 2 Temperature Read"
        # "Bay 1 Temperature Read"
        n918 = local read "Stop"() -> (w173:bool)
        n919 = call "IRSensorNIRead.vi"("error in (no error)"=w133, "Melexis_Cmmds"=w130, "Address"=u8 1, "device reference"=w152) -> ("error out"=w155:errorcluster, "Temperature"=w153:dbl, "device reference out"=w151:T6)  [unwired: 5 in]
        n920 = local write "error out"(w155) -> ()
        n921 = Unbundle By Name(w155) -> ("status"=w154:bool)
        n922 = call-poly <vilib>:"PID Control Input Filter.vi"("input"=w153) -> ("output"=w166:dbl)  [unwired: 4 in]
        n923 = case shown="False" w154 {
          tunnel: w165 -> [w182 _]
          tunnel: [w182 w183] -> w170
          frame False {
            n924 = local write "Temperature 1"(w182) -> ()
          }
          frame True {
            n925 = local read "Temperature 1"() -> (w183:dbl)
          }
        }
        n926 = flat-sequence {
          tunnel: w166 -> [w196]
          tunnel: [w196] -> w165
          tunnel: w151 -> [w195]
          tunnel: [w195] -> w150
          frame #0 {
            n927 = Wait (ms)(milliseconds to wait=u32 100) -> ()  [unwired: 1 out]
          }
        }
        n928 = call "IRSensorNIRead.vi"("error in (no error)"=w133, "Melexis_Cmmds"=w130, "Address"=u8 2, "device reference"=w150) -> ("error out"=w142:errorcluster, "Temperature"=w143:dbl, "device reference out"=w145:T6)  [unwired: 5 in]
        n929 = local write "error out"(w142) -> ()
        n930 = Unbundle By Name(w142) -> ("status"=w147:bool)
        n931 = call-poly <vilib>:"PID Control Input Filter.vi"("input"=w143) -> ("output"=w164:dbl)  [unwired: 4 in]
        n932 = case shown="True" w147 {
          tunnel: w163 -> [w180 _]
          tunnel: [w180 w181] -> w169
          frame False {
            n933 = local write "Temperature 2"(w180) -> ()
          }
          frame True {
            n934 = local read "Temperature 2"() -> (w181:dbl)
          }
        }
        n935 = flat-sequence {
          tunnel: w164 -> [w193]
          tunnel: [w193] -> w163
          tunnel: w145 -> [w192]
          tunnel: [w192] -> w144
          frame #0 {
            n936 = Wait (ms)(milliseconds to wait=u32 100) -> ()  [unwired: 1 out]
          }
        }
        n937 = call "IRSensorNIRead.vi"("error in (no error)"=w133, "Melexis_Cmmds"=w130, "Address"=u8 3, "device reference"=w144) -> ("error out"=w135:errorcluster, "Temperature"=w141:dbl, "device reference out"=w140:T6)  [unwired: 5 in]
        n938 = local write "error out"(w135) -> ()
        n939 = Unbundle By Name(w135) -> ("status"=w136:bool)
        n940 = case shown="False" w136 {
          tunnel: w160 -> [w178 _]
          tunnel: [w178 w179] -> w162
          frame False {
            n941 = local write "Temperature 3"(w178) -> ()
          }
          frame True {
            n942 = local read "Temperature 3"() -> (w179:dbl)
          }
        }
        n943 = call-poly <vilib>:"PID Control Input Filter.vi"("input"=w141) -> ("output"=w161:dbl)  [unwired: 4 in]
        n944 = flat-sequence {
          tunnel: w161 -> [w190]
          tunnel: [w190] -> w160
          tunnel: w140 -> [w189]
          tunnel: [w189] -> w138
          frame #0 {
            n945 = Wait (ms)(milliseconds to wait=u32 100) -> ()  [unwired: 1 out]
          }
        }
        n946 = call "IRSensorNIRead.vi"("error in (no error)"=w133, "Melexis_Cmmds"=w130, "Address"=u8 4, "device reference"=w138) -> ("error out"=w125:errorcluster, "Temperature"=w137:dbl, "device reference out"=w132:T6)  [unwired: 5 in]
        n947 = local write "error out"(w125) -> ()
        n948 = Unbundle By Name(w125) -> ("status"=w127:bool)
        n949 = case shown="True" w127 {
          tunnel: w158 -> [w176 _]
          tunnel: [w176 w177] -> w168
          frame False {
            n950 = local write "Temperature 4"(w176) -> ()
          }
          frame True {
            n951 = local read "Temperature 4"() -> (w177:dbl)
          }
        }
        n952 = call-poly <vilib>:"PID Control Input Filter.vi"("input"=w137) -> ("output"=w159:dbl)  [unwired: 4 in]
        n953 = flat-sequence {
          tunnel: w159 -> [w187]
          tunnel: [w187] -> w158
          tunnel: w132 -> [w186]
          tunnel: [w186] -> w131
          frame #0 {
            n954 = Wait (ms)(milliseconds to wait=u32 100) -> ()  [unwired: 1 out]
          }
        }
        n955 = call "IRSensorNIRead.vi"("error in (no error)"=w133, "Melexis_Cmmds"=w130, "Address"=u8 5, "device reference"=w131) -> ("error out"=w128:errorcluster, "Temperature"=w129:dbl)  [unwired: 5 in, 1 out]
        n956 = local write "error out"(w128) -> ()
        n957 = flat-sequence {
          tunnel: w157 -> [w184]
          tunnel: [w184] -> w156
          frame #0 {
            n958 = Wait (ms)(milliseconds to wait=u32 100) -> ()  [unwired: 1 out]
          }
        }
        n959 = Unbundle By Name(w128) -> ("status"=w126:bool)
        n960 = call-poly <vilib>:"PID Control Input Filter.vi"("input"=w129) -> ("output"=w157:dbl)  [unwired: 4 in]
        n961 = local write "error out"(w133) -> ()
        n962 = Build Array(w170, w169, w162, w168, w156) -> (w172:dbl[])
        n963 = Array To Cluster(array=w172) -> (cluster=→"Teperature Chart":T3)
        n964 = case shown="False" w126 {
          tunnel: w156 -> [w174 _]
          tunnel: [w174 w175] -> w167
          frame False {
            n965 = local write "Temperature 5"(w174) -> ()
          }
          frame True {
            n966 = local read "Temperature 5"() -> (w175:dbl)
          }
        }
        n967 = script code="MATLAB script"("T1"=w170, "T2"=w169, "T3"=w162, "T4"=w168, "T5"=w167) -> ()  [unwired: 1 in, 1 out]
      }
      n968 = while {
        stop <- w88 stop-if-true
        n969 = local read "Pump setpoint(ul/min) 1"() -> (w91:dbl)
        n970 = local read "Pump setpoint(ul/min) 2"() -> (w87:dbl)
        n971 = local read "Pump setpoint(ul/min) 3"() -> (w86:dbl)
        n972 = local read "Pump setpoint(ul/min) 4"() -> (w85:dbl)
        n973 = local read "Pump setpoint(ul/min) 5"() -> (w84:dbl)
        n974 = local read "Pump setpoint(ul/min) 6"() -> (w83:dbl)
        n975 = Build Array(w91, w87, w86, w85, w84, w83) -> (w92:dbl[])
        n976 = Array To Cluster(array=w92) -> (cluster=→"Pump Setpoints Chart":T3)
        n977 = Wait (ms)(milliseconds to wait=u32 5000) -> ()  [unwired: 1 out]
        n978 = local read "Stop"() -> (w88:bool)
      }
      n979 = while {
        stop <- w70 stop-if-true
        n980 = local read "System Error"() -> (w69:bool)
        n981 = Wait (ms)(milliseconds to wait=u32 300) -> ()  [unwired: 1 out]
        n982 = case shown="True" w69 {
          tunnel: [w74 w75] -> w67
          frame False {
            w71 = u16 2 items=["System  Error", "System Running", "System Standby"] ("System Status")
            w72 = u16 1 items=["System  Error", "System Running", "System Standby"] ("System Status")
            n983 = local read "running?"() -> (w73:bool)
            n984 = Select(t=w72, s=w73, f=w71) -> (s? t:f=w74:u16)
          }
          frame True {
            w75 = u16 0 items=["System  Error", "System Running", "System Standby"] ("System Status")
          }
        }
        n985 = local read "Stop"() -> (w70:bool)
        n986 = local write "System Status"(w67) -> ()
      }
      n987 = while {
        tunnel: w61 -> [w76]
        stop <- w82 stop-if-true
        n988 = call-poly <vilib>:"Analog Read.vi"("Analog Channel"=u8 0, "LINX Resource"=w76) -> ("Voltage"=w77:dbl)  [unwired: 6 in, 3 out]
        "Phase_Sensor_voltage" <- w77
        n989 = Wait (ms)(milliseconds to wait=u32 300) -> ()  [unwired: 1 out]
        n990 = Build Array(w77) -> (w79:dbl[])
        n991 = Array To Cluster(array=w79) -> (cluster=→"Phase Sensor Chart":T3)
        n992 = local read "Stop"() -> (w82:bool)
      }
      n993 = while {
        tunnel: w61 -> [w95]
        stop <- w120 stop-if-true
        w102 = 270
        w96 = 600
        w97 = 600
        # "Read Pressure and Flowrate"
        n994 = local read "Stop"() -> (w120:bool)
        n995 = call-poly <vilib>:"Analog Read.vi"("AI Channel(s)"=i32[] [14, 15, 14, 15], "LINX Resource"=w95) -> ("Voltages"=w93:dbl[])  [unwired: 6 in, 3 out]
        n996 = Index Array(array=w93, index=1) -> (element=w116:dbl)
        n997 = Index Array(array=w93, index=0) -> (element=w117:dbl)
        n998 = call-poly <vilib>:"PID Control Input Filter.vi"("input"=w116) -> ("output"=w109:dbl)  [unwired: 4 in]
        n999 = call-poly <vilib>:"PID Control Input Filter.vi"("input"=w117) -> ("output"=w108:dbl)  [unwired: 4 in]
        n1000 = Multiply(x=104.96 ("y"), y=w109) -> (x*y=w110:dbl)
        n1001 = Multiply(x=104.96 ("y"), y=w108) -> (x*y=w113:dbl)
        n1002 = Subtract(x=w110, y=24.077) -> (x-y=w100:dbl)
        n1003 = Subtract(x=w113, y=24.077) -> (x-y=w101:dbl)
        n1004 = Build Array(w97, w96) -> (w105:i32[])
        n1005 = Array To Cluster(array=w105) -> (cluster=→"Flowrate Chart":T4)
        n1006 = Build Array(w101, w100) -> (w106:dbl[])
        n1007 = local write "Flowrate Sensor 1"(w97) -> ()
        n1008 = local write "Flowrate Sensor 2"(w96) -> ()
        n1009 = local write "Pressure 1"(w101) -> ()
        n1010 = local write "Pressure 2"(w100) -> ()
        n1011 = Array To Cluster(array=w106) -> (cluster=→"Pressure Chart":T3)
        n1012 = Wait (ms)(milliseconds to wait=u32 500) -> ()  [unwired: 1 out]
        n1013 = script code="MATLAB script"("F1"=w97, "F2"=w96, "Pres1"=w101, "Pres2"=w100) -> ()  [unwired: 1 in, 1 out]
        n1014 = Greater?(x=w100, y=w102) -> (0:w98:bool)
        n1015 = Greater?(x=w101, y=w102) -> (0:w99:bool)
        n1016 = case shown="True" w99 {
          frame False {
          }
          frame True {
            w124 = TRUE ("Stop")
            n1017 = local write "System Error"(w124) -> ()
            n1018 = local write "Stop"(w124) -> ()
            n1019 = local write "Error Message"("Pressure Sensor 1 readings above 250psi") -> ()
            n1020 = script code="system_error = 1;"() -> ()  [unwired: 1 in, 1 out]
          }
        }
        n1021 = case shown="False" w98 {
          frame False {
          }
          frame True {
            w122 = TRUE ("Stop")
            n1022 = local write "System Error"(w122) -> ()
            n1023 = local write "Error Message"("Pressure Sensor 2 readings above 250psi") -> ()
            n1024 = local write "Stop"(w122) -> ()
            n1025 = script code="system_error = 1;"() -> ()  [unwired: 1 in, 1 out]
          }
        }
      }
    }
    frame #3 {
      # "Save and close xml and excel file"
      n1026 = script code="if exist('xl_file','var') & exist('xlApp','var')\n  xlWorkbook.SaveAs(xl_file);\n  xlWorkbook.Close;\n  xlApp.Quit;\n  xlApp.delete;\nend"() -> ()  [unwired: 1 in, 1 out]
    }
    frame #4 {
      w1380 = string[] ["e", "f", "g", "h", "i", "j"]
      # "End communication to hardware"
      n1027 = local read "Syringe_pump?"() -> (w1378:bool)
      n1028 = local read "COMM Port:: Harvard Syringe Pump"() -> (w1379:refnum<visa-resource-name>)
      n1029 = local read "IR Sensor Device"() -> (w1377:T6)
      n1030 = local read "COMM Port :: Milligat Pumps"() -> (w1382:refnum<visa-resource-name>)
      n1031 = call <vilib>:"Close.vi"("LINX Resource"=w1376) -> ()  [unwired: 10 in, 1 out]
      n1032 = Array Size(array=w1380) -> (size(s)=w1381:i32)
      n1033 = case shown="True" w1378 {
        tunnel: w1379 -> [_ w1383]
        frame False {
        }
        frame True {
          n1034 = call <instrlib>:"Stop Pump.vi"("VISA resource name"=w1383) -> ()  [unwired: 9 in, 2 out]
        }
      }
      n1035 = for {
        N: w1381 -> [_]
        tunnel: w1380 -> [w1384] mode=indexing
        tunnel: w1382 -> [w1385]
        n1036 = call "PumpStop.vi"("Pump Address"=w1384, "Pump COMM Port"=w1385) -> ()  [unwired: 9 in, 1 out]
        n1037 = Wait (ms)(milliseconds to wait=u32 300) -> ()  [unwired: 1 out]
      }
      n1038 = call-poly <vilib>:"NI-845x Close Reference.vi"("device reference"=w1377) -> ()  [unwired: 10 in, 1 out]
    }
    frame #5 {
      # "Display Error Messages if necessary"
      n1039 = local read "Error Message"() -> (w1387:string)
      n1040 = One Button Dialog(message=w1387) -> ()  [unwired: 1 in, 1 out]
    }
  }
